vi "gathering.vi"() -> ()   [LabVIEW 2016]
doc: "该模板用于创建生产者／消费者模式的应用程序，以事件驱动的方式，生成队列中的项。如需通过响应事件实现代码的异步执行，同时不影响用户界面的响应速度，可考虑用该模式替代“用户界面事件处理器”模式。"
panel:
  in  "Clear 2":bool
  in  "Clear":bool
  in  "控制选板":enum32{"主界面", "配置界面"}(tab)
  in  "设定压力":dbl
  in  "设定温度":dbl
  out "当前压力":dbl(knob) scale=0.0..10.0
  out "当前温度":dbl(slide) scale=0.0..100.0
  in  "刚度计算":bool
  out "样件结果数据":T1
  in  "自动":bool
  in  "手动":bool
  out "拉伸力":dbl
  in  "弯曲 2":bool caption="元素入队列"
  out "扭矩":dbl
  out "扭转角度2":dbl
  out "弯曲力":dbl
  out "拉伸位移":dbl
  out "扭转角度":dbl
  out "弯曲位移":dbl
  in  "复位3":bool caption="元素入队列"
  in  "拉伸":bool caption="元素入队列"
  in  "停止3":bool
  in  "复位2":bool caption="元素入队列"
  in  "扭转":bool caption="元素入队列"
  in  "停止2":bool
  in  "复位1":bool caption="元素入队列"
  in  "弯曲":bool caption="元素入队列"
  in  "停止1":bool
  out "弯曲":cluster{"Y":dbl[], "Y":dbl[]}[](graph)
  out "扭转":cluster{"Y":dbl[], "Y":dbl[]}[](graph)
  out "扭转刚度":dbl
  out "拉伸刚度":dbl
  out "弯曲刚度二":dbl
  out "弯曲刚度一":dbl
  out "拉伸":cluster{"Y":dbl[], "Y":dbl[]}[](graph)
  out "下行停止状态":bool
  out "下行状态":bool
  out "上行状态":bool
  out "上行停止状态":bool
  out "下行停止状态 2":bool
  out "下行状态 2":bool
  out "上行状态 2":bool
  out "上行停止状态 2":bool
  out "下行停止状态 3":bool
  out "下行状态 3":bool
  out "上行状态 3":bool
  out "上行停止状态 3":bool
  out "弯曲伺服":dbl
  out "扭转伺服":dbl
  out "拉伸伺服":dbl
  in  "设定弯曲行程":dbl=50000.0
  in  "设置弯曲速度":dbl=10000.0
  in  "设定扭转距离":dbl=50000.0
  in  "设置扭转速度":dbl=10000.0
  in  "设定拉升行程":dbl=50000.0
  in  "设置拉伸速度":dbl=10000.0
  in  "automitic":bool
  out "拉伸停止":bool
  out "扭转停止":bool
  out "弯曲停止":bool
  in  "运行状态 3":string
  in  "运行状态 2":string
  out "运行状态":string
  out "弯曲控制采集停止状态":bool
  in  "手动方向":bool
  in  "弯曲计算":string
  out "设备打开成功":bool
  out "私服使能关闭 3":bool
  in  "私服使能 3":bool
  out "改变速度成功 3":bool
  out "轴关闭成功 3":bool
  out "轴打开成功 3":bool
  out "急速停止成功 3":bool
  out "减速停止成功 3":bool
  out "相对运动 3":bool
  out "绝对运动 3":bool
  out "重置计数器成功 3":bool
  out "轴的状态: 3":string
  out "当前指令的速度 3":dbl
  out "私服使能关闭 2":bool
  in  "私服使能 2":bool
  out "改变速度成功 2":bool
  out "轴关闭成功 2":bool
  out "轴打开成功 2":bool
  out "急速停止成功 2":bool
  out "减速停止成功 2":bool
  out "相对运动 2":bool
  out "绝对运动 2":bool
  out "重置计数器成功 2":bool
  out "轴的状态: 2":string
  out "当前指令的速度 2":dbl
  out "当前轴达到最大速度":bool
  out "?":bool
  out "设备关闭成功":bool
  out "轴打开成功":bool
  out "急速停止成功":bool
  out "减速停止成功":bool
  out "重置计数器成功":bool
  in  "停止模式":enum32{"Dec", "Emg"}(radio)
  out "轴的数量":u32
  in  "Device Type":u16(ring) items=["PCI-1285 (M0)"]
  in  "withdraw":bool caption="停止"
  out "deviceList":u32[](array[numeric])
  out "DeviceHandle":u32
  out "AxisHandle_Array":u32[](array[numeric])
  in  "采集卡开关":bool=TRUE caption="stop(true)"
  out "error out":errorcluster
  out "轴的状态:":string
  # "控制状态"
  # "参数设置"
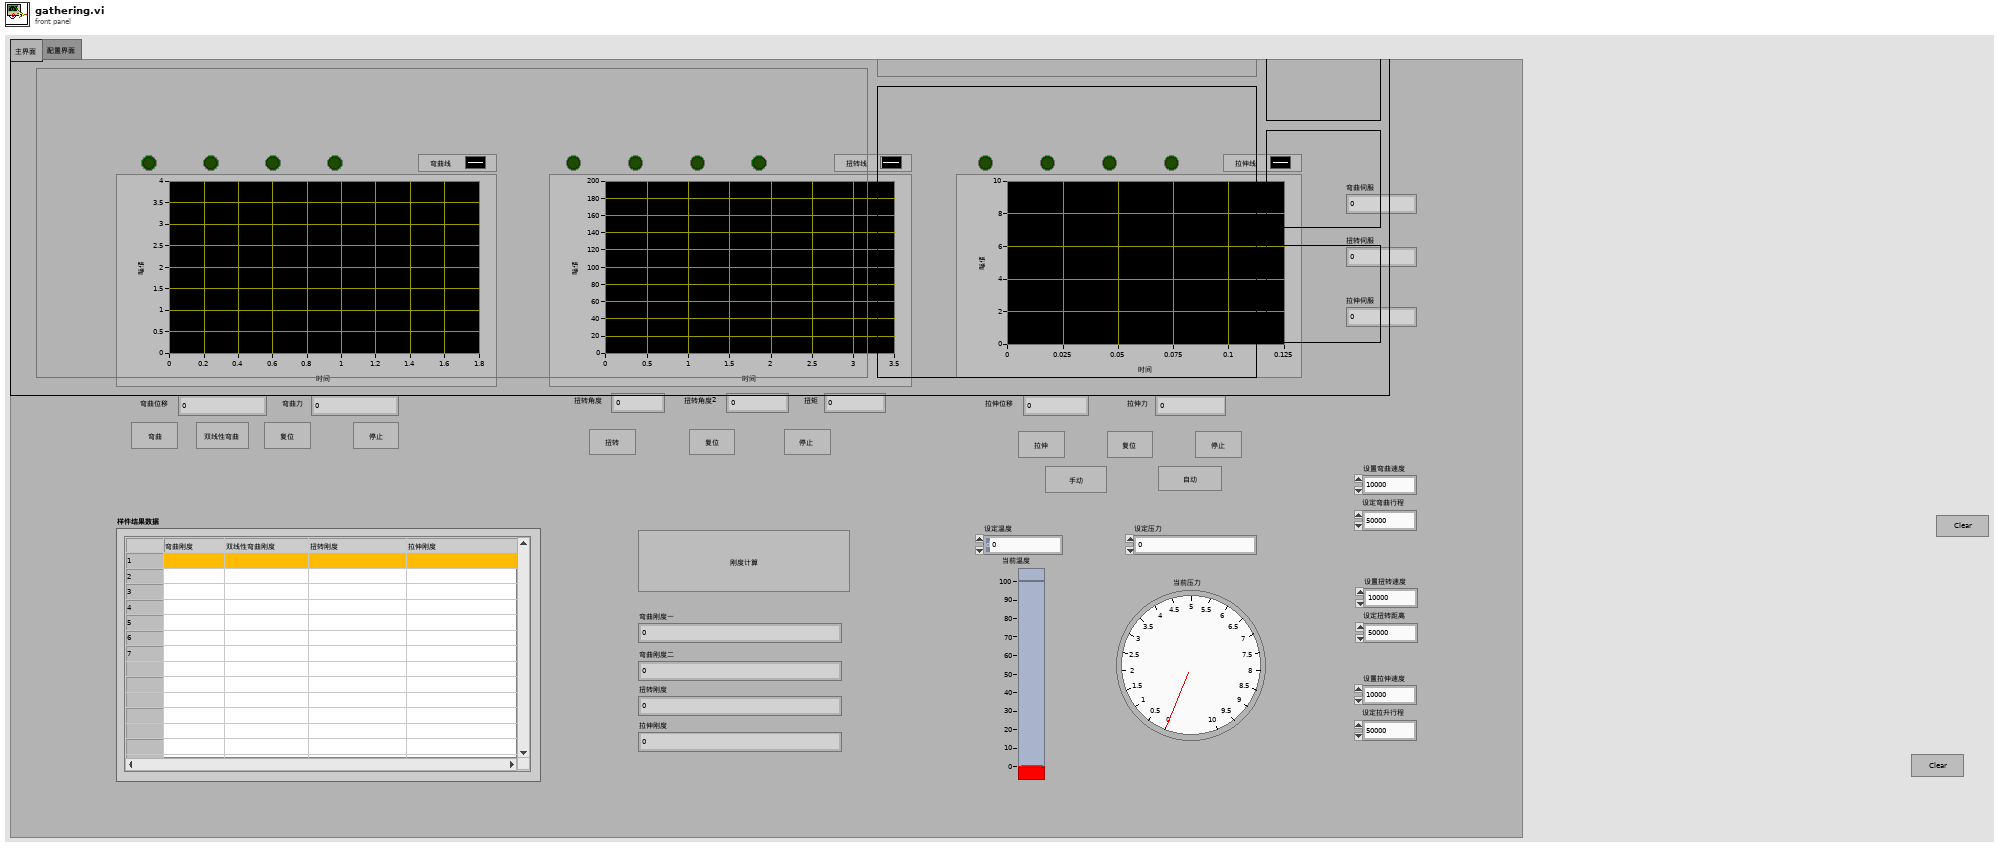
[diagram p1: front panel]
types:
  T1 = typedef "控件 1.ctl" = i32
  T2 = enum16{"open", "replace", "create", "open or create", "replace or create", "replace or create with confirmation"}
  T3 = enum8{"Enabled", "Disabled", "Disabled and Grayed Out"}
  T4 = cluster{"DeviceNum":u32, "U*8 Array":cluster{"U*8 Array[0]":u8, "U*8 Array[1]":u8, "U*8 Array[2]":u8, "U*8 Array[3]":u8, "U*8 Array[4]":u8, "U*8 Array[5]":u8, "U*8 Array[6]":u8, "U*8 Array[7]":u8, "U*8 Array[8]":u8, "U*8 Array[9]":u8, "U*8 Array[10]":u8, "U*8 Array[11]":u8, "U*8 Array[12]":u8, "U*8 Array[13]":u8, "U*8 Array[14]":u8, "U*8 Array[15]":u8, "U*8 Array[16]":u8, "U*8 Array[17]":u8, "U*8 Array[18]":u8, "U*8 Array[19]":u8, "U*8 Array[20]":u8, "U*8 Array[21]":u8, "U*8 Array[22]":u8, "U*8 Array[23]":u8, "U*8 Array[24]":u8, "U*8 Array[25]":u8, "U*8 Array[26]":u8, "U*8 Array[27]":u8, "U*8 Array[28]":u8, "U*8 Array[29]":u8, "U*8 Array[30]":u8, "U*8 Array[31]":u8, "U*8 Array[32]":u8, "U*8 Array[33]":u8, "U*8 Array[34]":u8, "U*8 Array[35]":u8, "U*8 Array[36]":u8, "U*8 Array[37]":u8, "U*8 Array[38]":u8, "U*8 Array[39]":u8, "U*8 Array[40]":u8, "U*8 Array[41]":u8, "U*8 Array[42]":u8, "U*8 Array[43]":u8, "U*8 Array[44]":u8, "U*8 Array[45]":u8, "U*8 Array[46]":u8, "U*8 Array[47]":u8, "U*8 Array[48]":u8, "U*8 Array[49]":u8}, "NumOfSubDevice":i16}[]
  T5 = cluster{"U*8 Array[0]":u8, "U*8 Array[1]":u8, "U*8 Array[2]":u8, "U*8 Array[3]":u8, "U*8 Array[4]":u8, "U*8 Array[5]":u8, "U*8 Array[6]":u8, "U*8 Array[7]":u8, "U*8 Array[8]":u8, "U*8 Array[9]":u8, "U*8 Array[10]":u8, "U*8 Array[11]":u8, "U*8 Array[12]":u8, "U*8 Array[13]":u8, "U*8 Array[14]":u8, "U*8 Array[15]":u8, "U*8 Array[16]":u8, "U*8 Array[17]":u8, "U*8 Array[18]":u8, "U*8 Array[19]":u8, "U*8 Array[20]":u8, "U*8 Array[21]":u8, "U*8 Array[22]":u8, "U*8 Array[23]":u8, "U*8 Array[24]":u8, "U*8 Array[25]":u8, "U*8 Array[26]":u8, "U*8 Array[27]":u8, "U*8 Array[28]":u8, "U*8 Array[29]":u8, "U*8 Array[30]":u8, "U*8 Array[31]":u8, "U*8 Array[32]":u8, "U*8 Array[33]":u8, "U*8 Array[34]":u8, "U*8 Array[35]":u8, "U*8 Array[36]":u8, "U*8 Array[37]":u8, "U*8 Array[38]":u8, "U*8 Array[39]":u8, "U*8 Array[40]":u8, "U*8 Array[41]":u8, "U*8 Array[42]":u8, "U*8 Array[43]":u8, "U*8 Array[44]":u8, "U*8 Array[45]":u8, "U*8 Array[46]":u8, "U*8 Array[47]":u8, "U*8 Array[48]":u8, "U*8 Array[49]":u8}
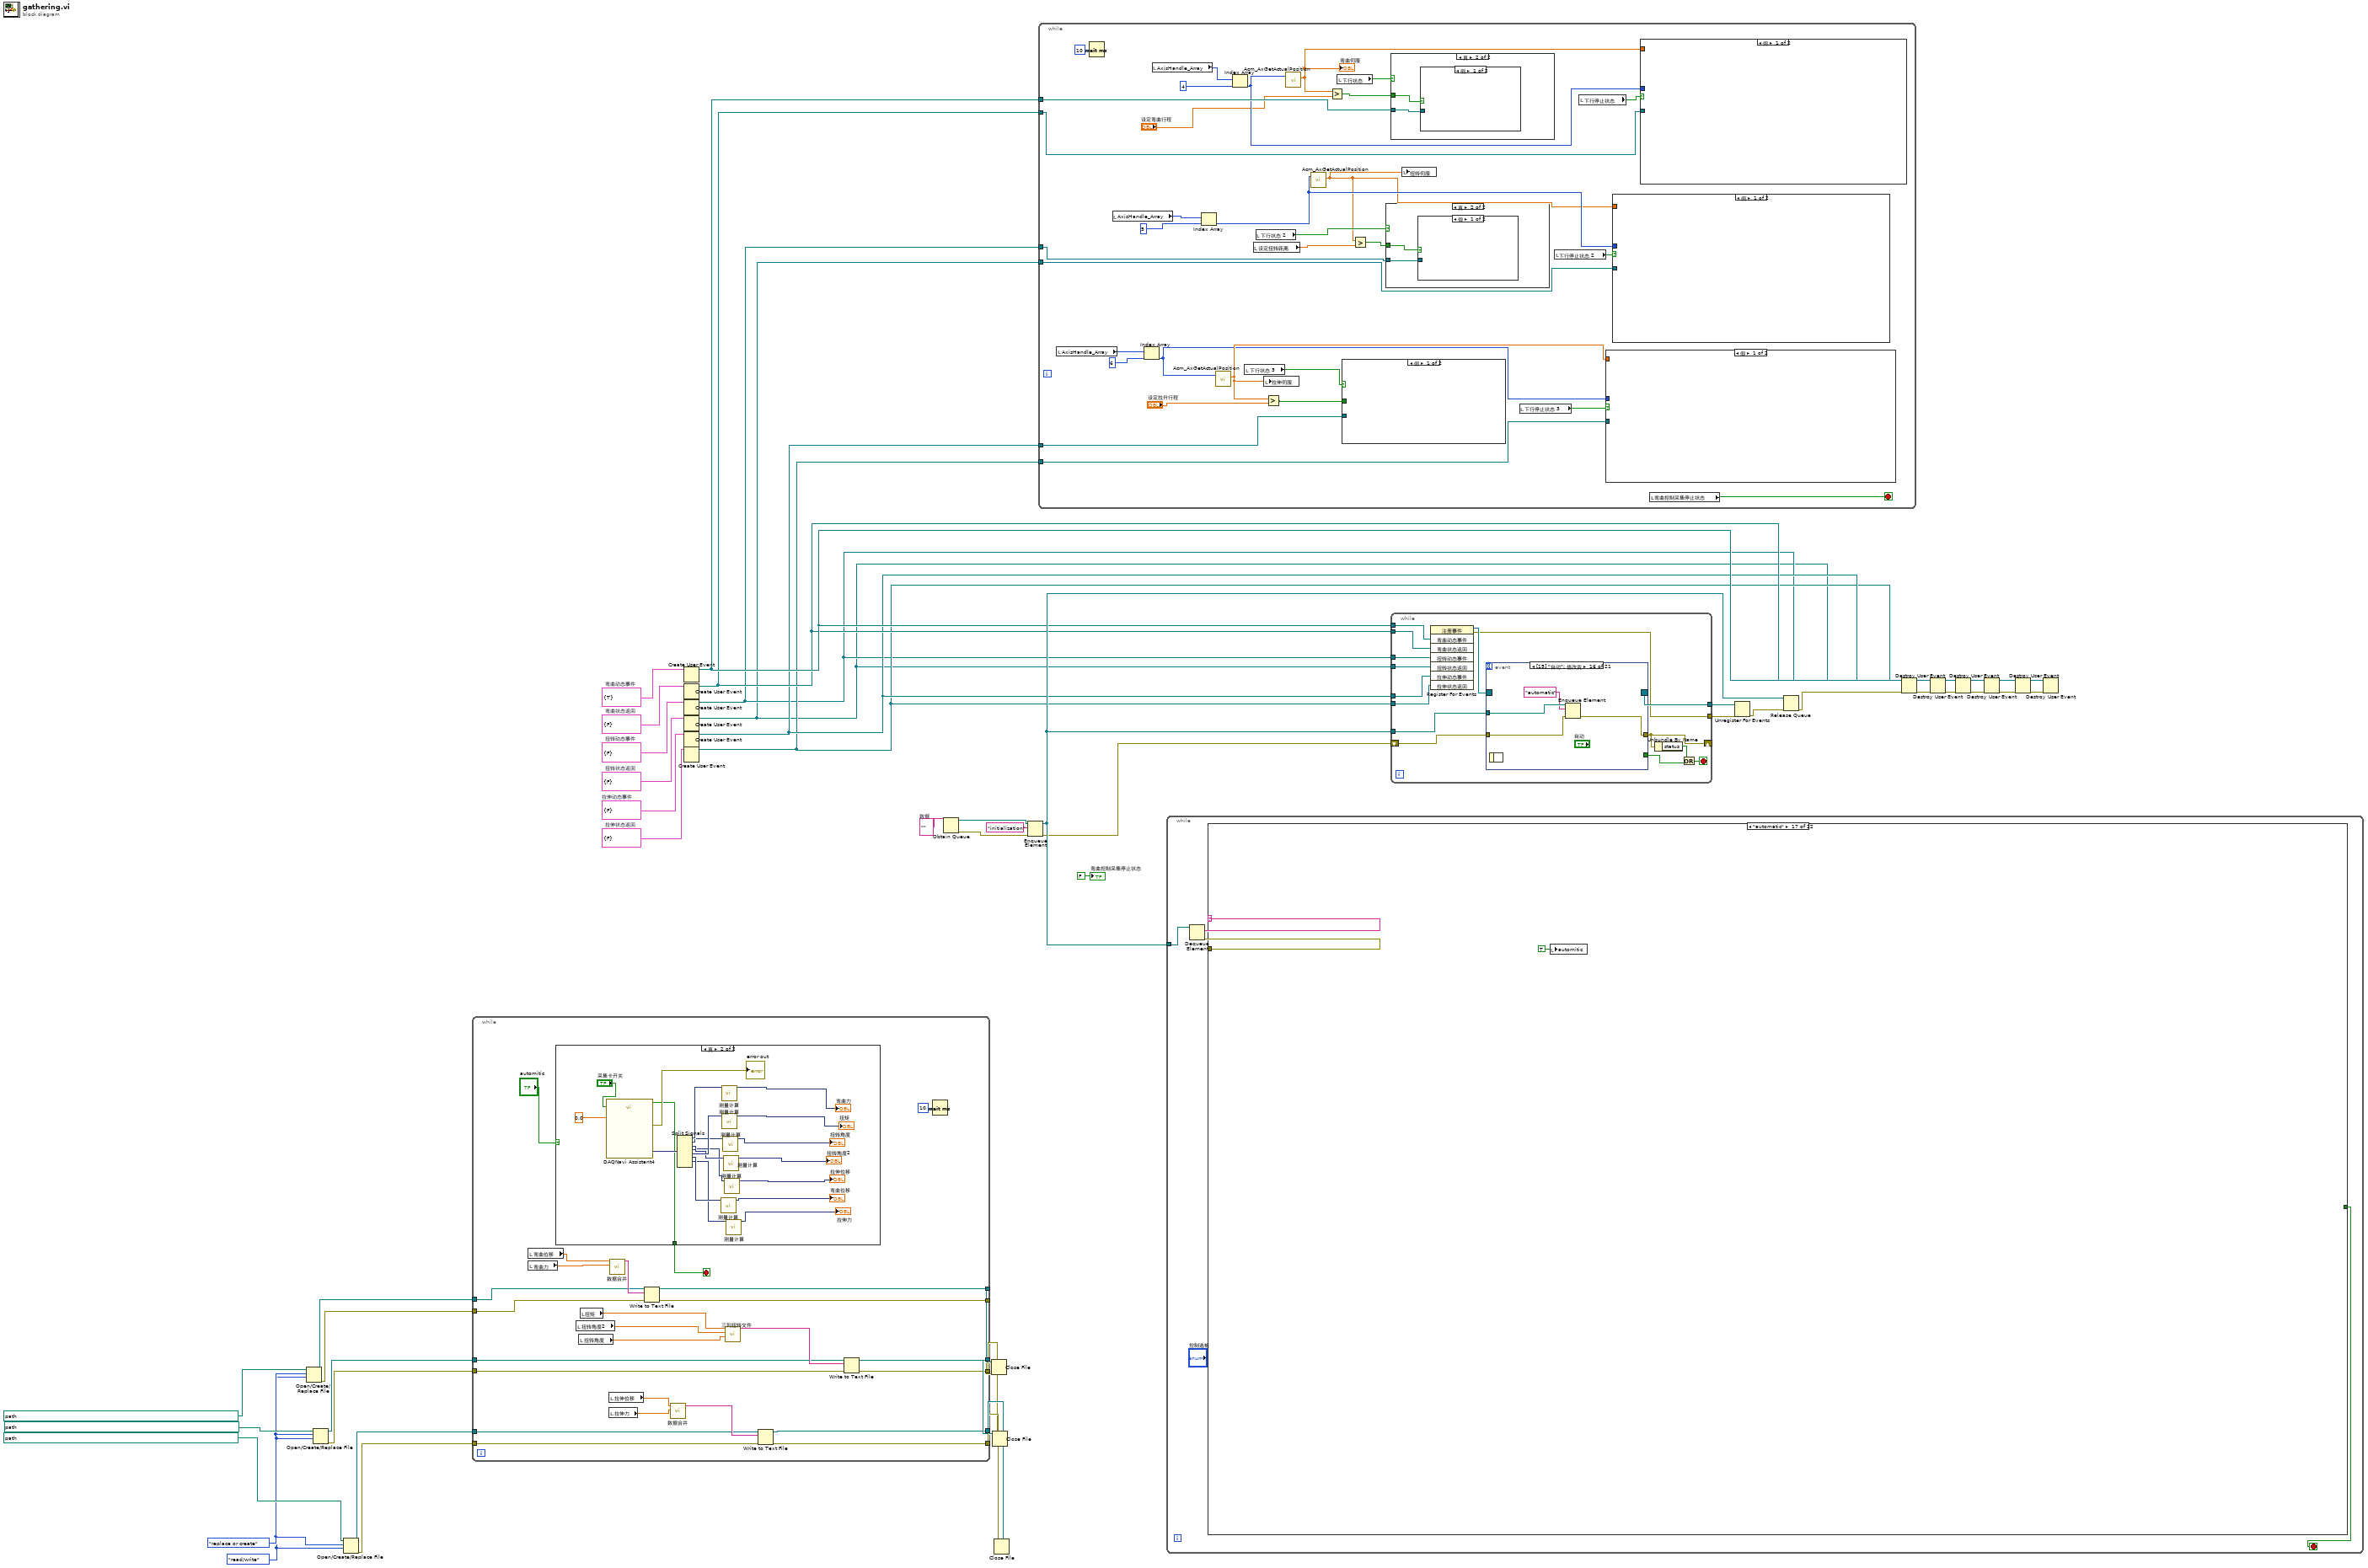
[diagram p0: block diagram]
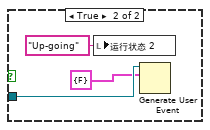
[diagram p3: hidden frame]
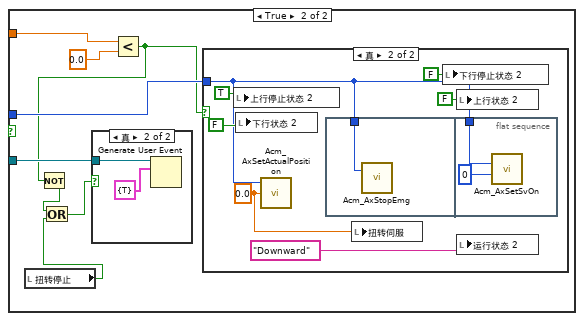
[diagram p4: hidden frame]
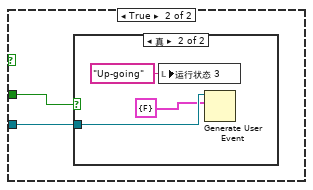
[diagram p7: hidden frame]
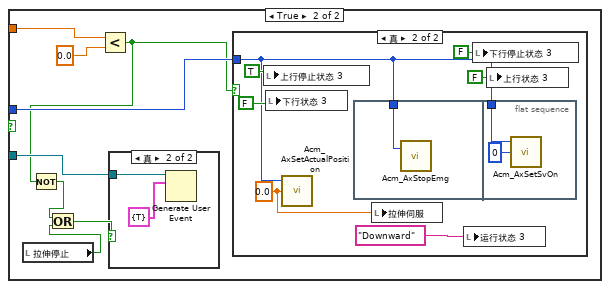
[diagram p9: hidden frame]
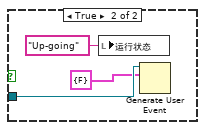
[diagram p13: hidden frame]
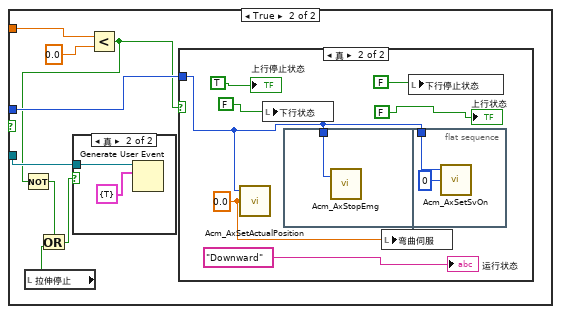
[diagram p14: hidden frame]
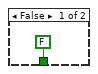
[diagram p17: hidden frame]
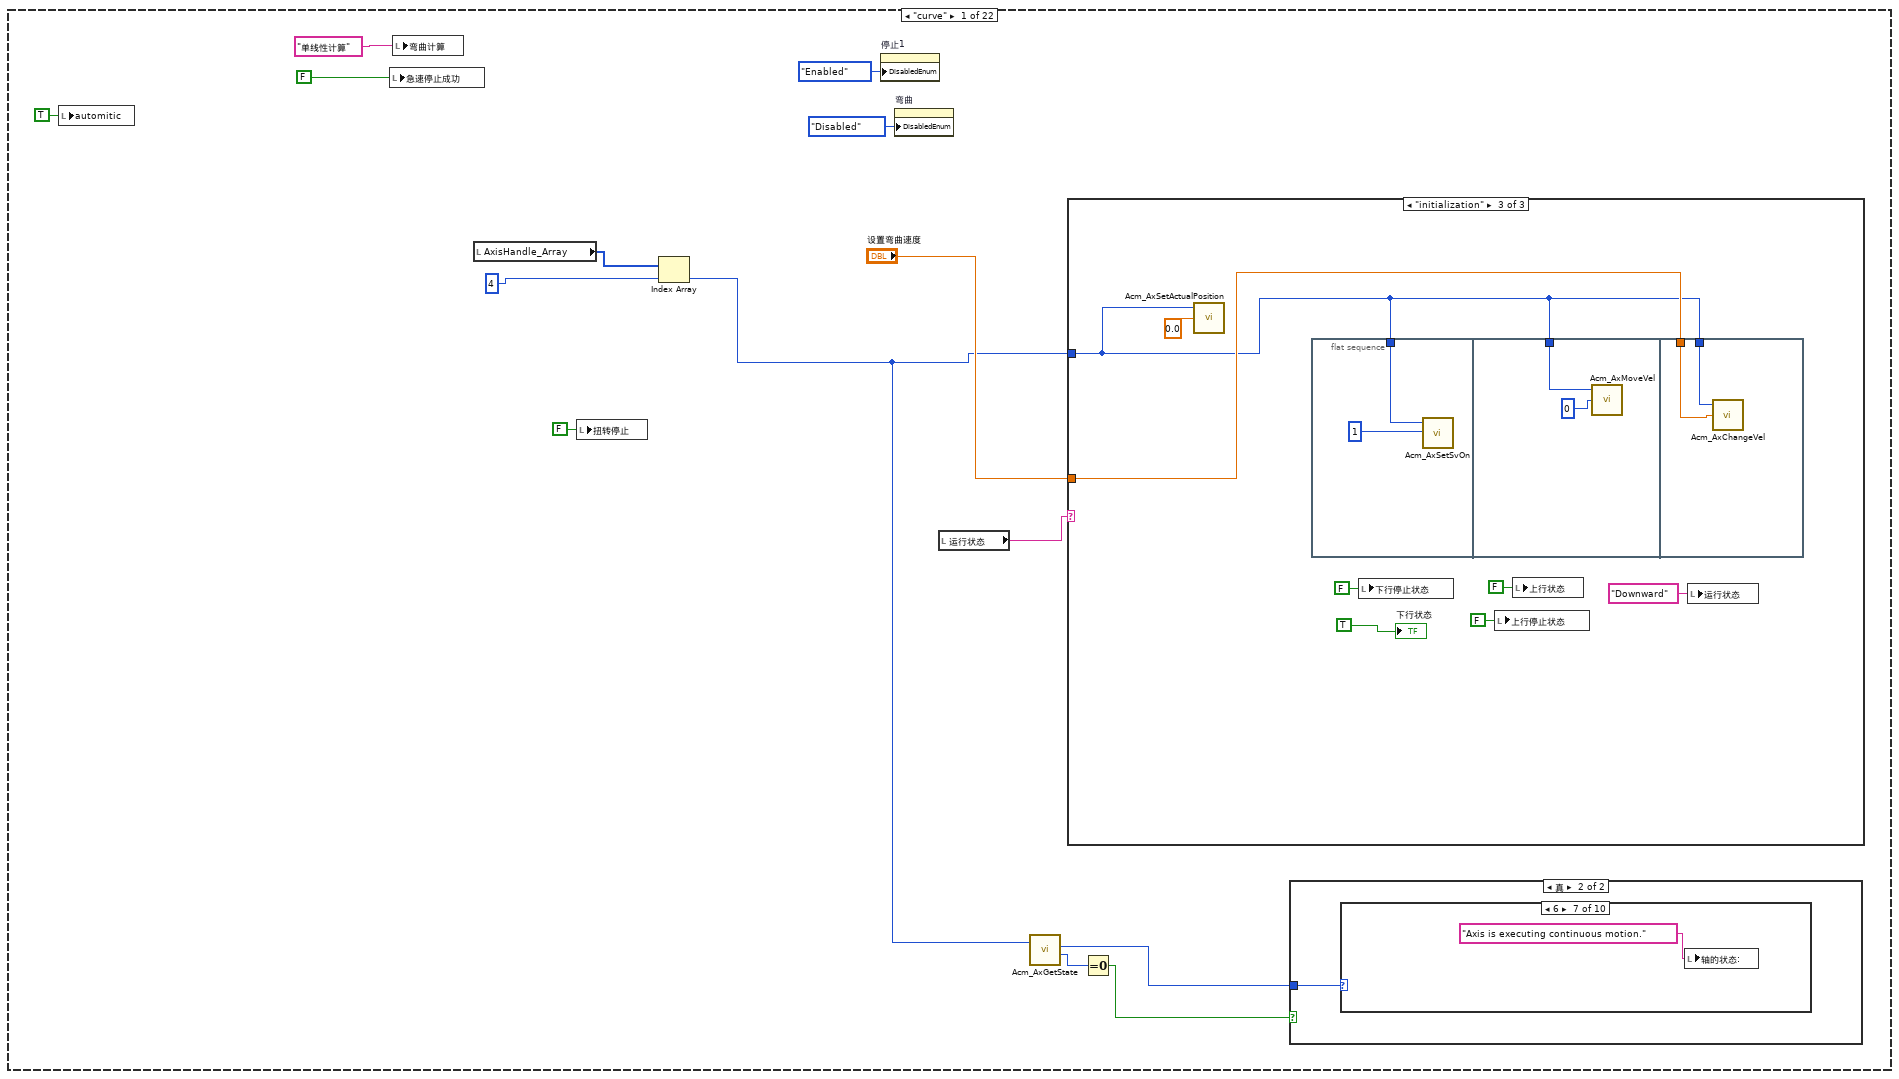
[diagram p18: hidden frame]
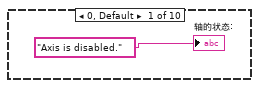
[diagram p20: hidden frame]
diagram:
  w14 = cluster{"拉升状态返回":bool} {"拉升状态返回"=FALSE}  # 拉伸状态返回
  w13 = cluster{"拉伸动态事件":bool} {"拉伸动态事件"=FALSE}  # 拉伸动态事件
  w12 = cluster{"扭转状态返回":bool} {"扭转状态返回"=FALSE}  # 扭转状态返回
  w11 = cluster{"扭转动态事件":bool} {"扭转动态事件"=FALSE}  # 扭转动态事件
  w16 = cluster{"弯曲状态返回":bool} {"弯曲状态返回"=FALSE}  # 弯曲状态返回
  w19 = cluster{"弯曲动态触发":bool} {"弯曲动态触发"=TRUE}  # 弯曲动态事件
  w33 = enum16{"read/write", "read-only", "write-only"}."read/write" ("权限(0:read/write)")
  w34 = T2."replace or create" ("操作(0:open)")
  w45 = ""  # 数据
  n1 = Open/Create/Replace File(file path (use dialog)=path "D:/controller/for_test_line/test_line/Collecting polymorphism/弯曲刚度检测数据.txt" ("文件路径（使用对话框）"), operation (0:open)=w34, access (0:read/write)=w33) -> (refnum out=w32:refnum<file>, error out=w31:errorcluster)  [unwired: 3 in, 1 out]
  n2 = Open/Create/Replace File(file path (use dialog)=path "D:/controller/for_test_line/test_line/Collecting polymorphism/扭转刚度检测数据.txt" ("文件路径（使用对话框）"), operation (0:open)=w34, access (0:read/write)=w33) -> (refnum out=w39:refnum<file>, error out=w38:errorcluster)  [unwired: 3 in, 1 out]
  n3 = Open/Create/Replace File(file path (use dialog)=path "D:/controller/for_test_line/test_line/Collecting polymorphism/拉伸刚度检测数据.txt" ("文件路径（使用对话框）"), operation (0:open)=w34, access (0:read/write)=w33) -> (refnum out=w37:refnum<file>, error out=w36:errorcluster)  [unwired: 3 in, 1 out]
  n4 = while {
    tunnel: w39 -> [w57]
    tunnel: w38 -> [w56]
    tunnel: w37 -> [w67]
    tunnel: w36 -> [w66]
    tunnel: w32 -> [w52]
    tunnel: w31 -> [w51]
    tunnel: [w65] -> w30
    tunnel: [w64] -> w29
    tunnel: [w54] -> w28
    tunnel: [w53] -> w27
    tunnel: [w50] -> w26
    tunnel: [w49] -> w25
    stop <- w46 stop-if-true
    n5 = local read "弯曲位移"() -> (w59:dbl)
    n6 = local read "弯曲力"() -> (w60:dbl)
    n7 = case shown="真" "automitic" {
      tunnel: [FALSE ("stopped") w72] -> w46
      frame False {
      }
      frame True {
        n8 = call "DAQNavi Assistant4"("stop(true)"="采集卡开关", "conversion rate(Hz)"=0.0) -> ("error out"=→"error out":errorcluster, "data out(DDT)"=w85:dynamicdata, "stopped"=w72:bool)  [unwired: 4 in, 19 out]
        n9 = Split Signals(w85) -> (w81:dynamicdata, w79:dynamicdata, w78:dynamicdata, w77:dynamicdata, w80:dynamicdata, w75:dynamicdata, w74:dynamicdata)  [unwired: 8 in, 1 out]
        n10 = call "测量计算.vi"("Dynamic Data输入"=w75) -> ("Dynamic Data输出"=→"弯曲位移":dynamicdata)  [unwired: 10 in]
        n11 = call "测量计算.vi"("Dynamic Data输入"=w81) -> ("Dynamic Data输出"=→"弯曲力":dynamicdata)  [unwired: 10 in]
        n12 = call "测量计算.vi"("Dynamic Data输入"=w80) -> ("Dynamic Data输出"=→"扭矩":dynamicdata)  [unwired: 10 in]
        n13 = call "测量计算.vi"("Dynamic Data输入"=w79) -> ("Dynamic Data输出"=→"扭转角度":dynamicdata)  [unwired: 10 in]
        n14 = call "测量计算.vi"("Dynamic Data输入"=w78) -> ("Dynamic Data输出"=→"扭转角度2":dynamicdata)  [unwired: 10 in]
        n15 = call "测量计算.vi"("Dynamic Data输入"=w77) -> ("Dynamic Data输出"=→"拉伸位移":dynamicdata)  [unwired: 10 in]
        n16 = call "测量计算.vi"("Dynamic Data输入"=w74) -> ("Dynamic Data输出"=→"拉伸力":dynamicdata)  [unwired: 10 in]
      }
    }
    n17 = local read "扭转角度2"() -> (w62:dbl)
    n18 = local read "扭转角度"() -> (w61:dbl)
    n19 = local read "扭矩"() -> (w63:dbl)
    n20 = local read "拉伸位移"() -> (w69:dbl)
    n21 = local read "拉伸力"() -> (w70:dbl)
    n22 = call "数据合并.vi"("数值输入"=w60, "数值 3"=w59) -> ("字符串"=w55:string)  [unwired: 9 in]
    n23 = Write to Text File(file (use dialog)=w52, text=w55, error in=w51) -> (refnum out=w50:refnum<file>, error out=w49:errorcluster)  [unwired: 1 in, 1 out]
    n24 = call "数据合并.vi"("数值输入"=w70, "数值 3"=w69) -> ("字符串"=w68:string)  [unwired: 9 in]
    n25 = call "三列扭转文件.vi"("扭转角度"=w61, "扭转角度2"=w62, "扭矩"=w63) -> ("字符串"=w58:string)  [unwired: 8 in]
    n26 = Write to Text File(file (use dialog)=w67, text=w68, error in=w66) -> (refnum out=w65:refnum<file>, error out=w64:errorcluster)  [unwired: 1 in, 1 out]
    n27 = Write to Text File(file (use dialog)=w57, text=w58, error in=w56) -> (refnum out=w54:refnum<file>, error out=w53:errorcluster)  [unwired: 1 in, 1 out]
    n28 = Wait (ms)(milliseconds to wait=u32 10 ("等待时间（毫秒）")) -> ()  [unwired: 1 out]
  }
  n29 = Create User Event(user event datatype=w19) -> (user event=w20:refnum<user-event>)  [unwired: 1 in, 1 out]
  n30 = Create User Event(user event datatype=w16) -> (user event=w17:refnum<user-event>)  [unwired: 1 in, 1 out]
  n31 = Create User Event(user event datatype=w11) -> (user event=w4:refnum<user-event>)  [unwired: 1 in, 1 out]
  n32 = Create User Event(user event datatype=w12) -> (user event=w3:refnum<user-event>)  [unwired: 1 in, 1 out]
  n33 = Create User Event(user event datatype=w13) -> (user event=w6:refnum<user-event>)  [unwired: 1 in, 1 out]
  n34 = Create User Event(user event datatype=w14) -> (user event=w5:refnum<user-event>)  [unwired: 1 in, 1 out]
  n35 = Obtain Queue(element data type=w45) -> (queue out=w44:refnum<queue>, error out=w43:errorcluster)  [unwired: 4 in, 1 out]
  n36 = Close File(refnum=w26, error in=w25) -> ()  [unwired: 2 out]
  n37 = Close File(refnum=w28, error in=w27) -> ()  [unwired: 2 out]
  n38 = Close File(refnum=w30, error in=w29) -> ()  [unwired: 2 out]
  n39 = Enqueue Element(queue=w44, element="initialization" ("元素"), error in (no error)=w43) -> (queue out=w24:refnum<queue>, error out=w15:errorcluster)  [unwired: 1 in, 1 out]
  n40 = while "While循环" {
    tunnel: w20 -> [w119]
    tunnel: w17 -> [w117]
    tunnel: w6 -> [w106]
    tunnel: w5 -> [w105]
    tunnel: w4 -> [w96]
    tunnel: w3 -> [w95]
    stop <- w120 stop-if-true
    # "弯曲位置采集"
    n41 = local read "AxisHandle_Array"() -> (w108:u32[])
    n42 = Wait (ms)(milliseconds to wait=u32 10 ("等待时间（毫秒）")) -> ()  [unwired: 1 out]
    n43 = local read "AxisHandle_Array"() -> (w103:u32[])
    n44 = Index Array(array=w108, index=6 ("索引")) -> (element=w110:u32)
    n45 = local read "AxisHandle_Array"() -> (w121:u32[])
    n46 = Index Array(array=w103, index=5 ("索引")) -> (element=w101:u32)
    n47 = call <userlib>:"Acm_AxGetActualPosition.vi"("AxisHandle"=w110) -> ("Position"=w112:dbl)  [unwired: 1 in, 3 out]
    n48 = Index Array(array=w121, index=4 ("索引")) -> (element=w116:u32)
    n49 = local read "下行状态 3"() -> (w111:bool)
    n50 = local read "设定扭转距离"() -> (w98:dbl)
    n51 = local read "下行状态 2"() -> (w100:bool)
    n52 = local write "拉伸伺服"(w112) -> ()
    n53 = Greater?(x=w112, y="设定拉升行程") -> (0:w113:bool)
    n54 = call <userlib>:"Acm_AxGetActualPosition.vi"("AxisHandle"=w116) -> ("Position"=w91:dbl)  [unwired: 1 in, 3 out]
    "弯曲伺服" <- w91
    n55 = call <userlib>:"Acm_AxGetActualPosition.vi"("AxisHandle"=w101) -> ("Position"=w99:dbl)  [unwired: 1 in, 3 out]
    n56 = Greater?(x=w91, y="设定弯曲行程") -> (0:w114:bool)
    n57 = local read "下行状态"() -> (w115:bool)
    n58 = case shown="假" w111 {
      tunnel: w113 -> [_ w149]
      tunnel: w106 -> [_ w148]
      frame False {
      }
      frame True {
        n59 = case shown="真" w149 {
          tunnel: w148 -> [_ w152]
          frame False {
          }
          frame True {
            n60 = local write "运行状态 3"("Up-going" ("运行状态")) -> ()
            n61 = Generate User Event(user event=w152, event data cluster=cluster{"弯曲动态触发":bool} {"弯曲动态触发"=FALSE} ("事件数据")) -> ()  [unwired: 2 in, 2 out]
          }
        }
      }
    }
    n62 = Greater?(x=w99, y=w98) -> (0:w97:bool)
    n63 = case shown="真" w100 {
      tunnel: w97 -> [_ w124]
      tunnel: w96 -> [_ w123]
      frame False {
      }
      frame True {
        n64 = case shown="假" w124 {
          tunnel: w123 -> [_ w127]
          frame False {
          }
          frame True {
            n65 = local write "运行状态 2"("Up-going" ("运行状态")) -> ()
            n66 = Generate User Event(user event=w127, event data cluster=cluster{"弯曲动态触发":bool} {"弯曲动态触发"=FALSE} ("事件数据")) -> ()  [unwired: 2 in, 2 out]
          }
        }
      }
    }
    n67 = case shown="真" w115 {
      tunnel: w114 -> [_ w174]
      tunnel: w119 -> [_ w173]
      frame False {
      }
      frame True {
        n68 = case shown="假" w174 {
          tunnel: w173 -> [_ w177]
          frame False {
          }
          frame True {
            n69 = local write "运行状态"("Up-going" ("运行状态")) -> ()
            n70 = Generate User Event(user event=w177, event data cluster=cluster{"弯曲动态触发":bool} {"弯曲动态触发"=FALSE} ("事件数据")) -> ()  [unwired: 2 in, 2 out]
          }
        }
      }
    }
    n71 = local write "扭转伺服"(w99) -> ()
    n72 = local read "下行停止状态 3"() -> (w109:bool)
    n73 = local read "下行停止状态 2"() -> (w102:bool)
    n74 = local read "下行停止状态"() -> (w118:bool)
    n75 = case shown="假" w109 {
      tunnel: w105 -> [_ w160]
      tunnel: w112 -> [_ w159]
      tunnel: w110 -> [_ w157]
      frame False {
      }
      frame True {
        n76 = local read "拉伸停止"() -> (w154:bool)
        n77 = Less?(x=w159, y=0.0) -> (x < y?=w156:bool)
        n78 = Not(x=w156) -> (.not. x?=w155:bool)
        n79 = Or(x=w155, y=w154) -> (x .or. y?=w153:bool)
        n80 = case shown="真" w153 {
          tunnel: w160 -> [_ w162]
          frame False {
          }
          frame True {
            n81 = Generate User Event(user event=w162, event data cluster=cluster{"弯曲动态触发":bool} {"弯曲动态触发"=TRUE} ("事件数据")) -> ()  [unwired: 2 in, 2 out]
          }
        }
        n82 = case shown="真" w156 {
          tunnel: w157 -> [_ w165]
          frame False {
          }
          frame True {
            w164 = 0.0 ("Position")
            n83 = local write "上行停止状态 3"(TRUE ("上行停止状态")) -> ()
            n84 = local write "下行状态 3"(FALSE ("下行状态")) -> ()
            n85 = call <userlib>:"Acm_AxSetActualPosition.vi"("Position"=w164, "AxisHandle"=w165) -> ()  [unwired: 1 in, 3 out]
            n86 = flat-sequence {
              tunnel: w165 -> [w170]
              tunnel: w165 -> [w172]
              frame #0 {
                n87 = call <userlib>:"Acm_AxStopEmg.vi"("AxisHandle"=w170) -> ()  [unwired: 1 in, 3 out]
              }
              frame #1 {
                n88 = call <userlib>:"Acm_AxSetSvOn.vi"("OnOff"=u32 0, "AxisHandle"=w172) -> ()  [unwired: 1 in, 3 out]
              }
            }
            n89 = local write "拉伸伺服"(w164) -> ()
            n90 = local write "运行状态 3"("Downward" ("运行状态 3")) -> ()
            n91 = local write "下行停止状态 3"(FALSE ("下行停止状态")) -> ()
            n92 = local write "上行状态 3"(FALSE ("上行状态")) -> ()
          }
        }
      }
    }
    n93 = case shown="假" w102 {
      tunnel: w95 -> [_ w135]
      tunnel: w99 -> [_ w134]
      tunnel: w101 -> [_ w132]
      frame False {
      }
      frame True {
        n94 = local read "扭转停止"() -> (w130:bool)
        n95 = Less?(x=w134, y=0.0) -> (x < y?=w131:bool)
        n96 = Not(x=w131) -> (.not. x?=w129:bool)
        n97 = Or(x=w129, y=w130) -> (x .or. y?=w128:bool)
        n98 = case shown="真" w128 {
          tunnel: w135 -> [_ w137]
          frame False {
          }
          frame True {
            n99 = Generate User Event(user event=w137, event data cluster=cluster{"弯曲动态触发":bool} {"弯曲动态触发"=TRUE} ("事件数据")) -> ()  [unwired: 2 in, 2 out]
          }
        }
        n100 = case shown="真" w131 {
          tunnel: w132 -> [_ w140]
          frame False {
          }
          frame True {
            w139 = 0.0 ("Position")
            n101 = local write "上行停止状态 2"(TRUE ("上行停止状态")) -> ()
            n102 = local write "下行状态 2"(FALSE ("下行状态")) -> ()
            n103 = call <userlib>:"Acm_AxSetActualPosition.vi"("Position"=w139, "AxisHandle"=w140) -> ()  [unwired: 1 in, 3 out]
            n104 = flat-sequence {
              tunnel: w140 -> [w145]
              tunnel: w140 -> [w147]
              frame #0 {
                n105 = call <userlib>:"Acm_AxStopEmg.vi"("AxisHandle"=w145) -> ()  [unwired: 1 in, 3 out]
              }
              frame #1 {
                n106 = call <userlib>:"Acm_AxSetSvOn.vi"("OnOff"=u32 0, "AxisHandle"=w147) -> ()  [unwired: 1 in, 3 out]
              }
            }
            n107 = local write "扭转伺服"(w139) -> ()
            n108 = local write "下行停止状态 2"(FALSE ("下行停止状态")) -> ()
            n109 = local write "上行状态 2"(FALSE ("上行状态")) -> ()
            n110 = local write "运行状态 2"("Downward" ("运行状态 2")) -> ()
          }
        }
      }
    }
    n111 = case shown="假" w118 {
      tunnel: w117 -> [_ w185]
      tunnel: w91 -> [_ w184]
      tunnel: w116 -> [_ w182]
      frame False {
      }
      frame True {
        n112 = local read "拉伸停止"() -> (w180:bool)
        n113 = Less?(x=w184, y=0.0) -> (x < y?=w181:bool)
        n114 = Not(x=w181) -> (.not. x?=w179:bool)
        n115 = Or(x=w179, y=w180) -> (x .or. y?=w178:bool)
        n116 = case shown="真" w178 {
          tunnel: w185 -> [_ w187]
          frame False {
          }
          frame True {
            n117 = Generate User Event(user event=w187, event data cluster=cluster{"弯曲动态触发":bool} {"弯曲动态触发"=TRUE} ("事件数据")) -> ()  [unwired: 2 in, 2 out]
          }
        }
        n118 = case shown="真" w181 {
          tunnel: w182 -> [_ w192]
          frame False {
          }
          frame True {
            w191 = 0.0 ("Position")
            n119 = call <userlib>:"Acm_AxSetActualPosition.vi"("Position"=w191, "AxisHandle"=w192) -> ()  [unwired: 1 in, 3 out]
            n120 = local write "下行状态"(FALSE ("下行状态")) -> ()
            n121 = flat-sequence {
              tunnel: w192 -> [w195]
              tunnel: w192 -> [w197]
              frame #0 {
                n122 = call <userlib>:"Acm_AxStopEmg.vi"("AxisHandle"=w195) -> ()  [unwired: 1 in, 3 out]
              }
              frame #1 {
                n123 = call <userlib>:"Acm_AxSetSvOn.vi"("OnOff"=u32 0, "AxisHandle"=w197) -> ()  [unwired: 1 in, 3 out]
              }
            }
            n124 = local write "弯曲伺服"(w191) -> ()
            n125 = local write "下行停止状态"(FALSE ("下行停止状态")) -> ()
            "运行状态" <- "Downward" ("运行状态")
            "上行状态" <- FALSE ("上行状态")
            "上行停止状态" <- TRUE ("上行停止状态")
          }
        }
      }
    }
    n126 = local read "弯曲控制采集停止状态"() -> (w120:bool)
  }
  n127 = while {
    tunnel: w24 -> [w201]
    stop <- w200 stop-if-true
    n128 = Dequeue Element(queue=w201) -> (element=w199:string, error out=w198:errorcluster)  [unwired: 2 in, 2 out]
    n129 = case shown="\"automatic\"" w199 {
      tunnel: [_ _ _ _ FALSE ("status") _ _ _ _ _ _ _ _ _ _ _ _ _ _ _ w873 w909] -> w200
      tunnel: w198 -> [_ _ _ _ _ _ _ _ _ _ _ _ _ _ _ _ _ _ _ _ w875 w911]
      frame "curve" {
        n130 = local write "automitic"(TRUE ("automitic")) -> ()
        n131 = local write "急速停止成功"(FALSE ("急速停止成功")) -> ()
        n132 = local write "弯曲计算"("单线性计算" ("采集状态")) -> ()
        n133 = local read "AxisHandle_Array"() -> (w214:u32[])
        n134 = local write "扭转停止"(FALSE ("扭转停止")) -> ()
        n135 = Index Array(array=w214, index=4 ("索引")) -> (element=w206:u32)
        n136 = property on="停止1" class="Bool"("DisabledEnum"=T3."Enabled" ("禁用")) -> ()  [unwired: 2 in, 2 out]
        n137 = property on="弯曲" class="Bool"("DisabledEnum"=T3."Disabled" ("禁用")) -> ()  [unwired: 2 in, 2 out]
        n138 = local read "运行状态"() -> (w211:string)
        n139 = call <userlib>:"Acm_AxGetState.vi"("AxisHandle"=w206) -> ("ReturnValue"=w210:u32, "Status"=w208:u16)  [unwired: 1 in, 2 out]
        n140 = case shown="\"initialization\"" w211 {
          tunnel: w206 -> [w229 w242 w253]
          tunnel: "设置弯曲速度" -> [w228 w241 w260]
          frame "Downward", Default {
            n141 = flat-sequence {
              tunnel: w229 -> [w234]
              tunnel: w229 -> [w237]
              tunnel: w229 -> [w239]
              tunnel: w228 -> [w238]
              frame #0 {
                n142 = call <userlib>:"Acm_AxSetSvOn.vi"("OnOff"=u32 1, "AxisHandle"=w234) -> ()  [unwired: 1 in, 3 out]
              }
              frame #1 {
                n143 = call <userlib>:"Acm_AxMoveVel.vi"("Direction"=u16 0, "AxisHandle"=w237) -> ()  [unwired: 1 in, 3 out]
              }
              frame #2 {
                n144 = call <userlib>:"Acm_AxChangeVel.vi"("NewVelocity"=w238, "AxisHandle"=w239) -> ()  [unwired: 1 in, 3 out]
              }
            }
            n145 = local write "下行停止状态"(FALSE ("下行停止状态")) -> ()
            n146 = local write "下行状态"(TRUE ("下行状态")) -> ()
            n147 = local write "上行停止状态"(FALSE ("上行停止状态")) -> ()
            n148 = local write "上行状态"(FALSE ("上行状态")) -> ()
            n149 = local write "运行状态"("Downward" ("运行状态")) -> ()
          }
          frame "Up-going" {
            n150 = flat-sequence {
              tunnel: w242 -> [w247]
              tunnel: w242 -> [w249]
              tunnel: w242 -> [w252]
              tunnel: w241 -> [w251]
              frame #0 {
                n151 = call <userlib>:"Acm_AxSetSvOn.vi"("OnOff"=u32 1, "AxisHandle"=w247) -> ()  [unwired: 1 in, 3 out]
              }
              frame #1 {
                n152 = call <userlib>:"Acm_AxMoveVel.vi"("Direction"=u16 1, "AxisHandle"=w249) -> ()  [unwired: 1 in, 3 out]
              }
              frame #2 {
                n153 = call <userlib>:"Acm_AxChangeVel.vi"("NewVelocity"=w251, "AxisHandle"=w252) -> ()  [unwired: 1 in, 3 out]
              }
            }
            n154 = local write "下行停止状态"(TRUE ("下行停止状态")) -> ()
            n155 = local write "下行状态"(FALSE ("下行状态")) -> ()
            n156 = local write "上行状态"(TRUE ("上行状态")) -> ()
            n157 = local write "上行停止状态"(FALSE ("上行停止状态")) -> ()
            n158 = local write "运行状态"("Up-going" ("运行状态")) -> ()
          }
          frame "initialization" {
            n159 = call <userlib>:"Acm_AxSetActualPosition.vi"("Position"=0.0, "AxisHandle"=w253) -> ()  [unwired: 1 in, 3 out]
            n160 = flat-sequence {
              tunnel: w253 -> [w261]
              tunnel: w253 -> [w263]
              tunnel: w253 -> [w266]
              tunnel: w260 -> [w265]
              frame #0 {
                n161 = call <userlib>:"Acm_AxSetSvOn.vi"("OnOff"=u32 1, "AxisHandle"=w261) -> ()  [unwired: 1 in, 3 out]
              }
              frame #1 {
                n162 = call <userlib>:"Acm_AxMoveVel.vi"("Direction"=u16 0, "AxisHandle"=w263) -> ()  [unwired: 1 in, 3 out]
              }
              frame #2 {
                n163 = call <userlib>:"Acm_AxChangeVel.vi"("NewVelocity"=w265, "AxisHandle"=w266) -> ()  [unwired: 1 in, 3 out]
              }
            }
            n164 = local write "下行停止状态"(FALSE ("下行停止状态")) -> ()
            n165 = local write "上行停止状态"(FALSE ("上行停止状态")) -> ()
            n166 = local write "上行状态"(FALSE ("上行状态")) -> ()
            n167 = local write "运行状态"("Downward" ("运行状态")) -> ()
            "下行状态" <- TRUE ("下行状态")
          }
        }
        n168 = Equal To 0?(x=w210) -> (x = 0?=w207:bool)
        n169 = case shown="真" w207 {
          tunnel: w208 -> [_ w216]
          frame False {
          }
          frame True {
            n170 = case shown="6" w216 {
              frame 0, Default {
                "轴的状态:" <- "Axis is disabled." ("Axis State:")
              }
              frame 1 {
                n171 = local write "轴的状态:"("Axis is ready." ("Axis State:")) -> ()
              }
              frame 2 {
                n172 = local write "轴的状态:"("Axis is stopping." ("Axis State:")) -> ()
              }
              frame 3 {
                n173 = local write "轴的状态:"("Axis is Error_Stopped." ("Axis State:")) -> ()
              }
              frame 4 {
                n174 = local write "轴的状态:"("Axis is executing home motion." ("Axis State:")) -> ()
              }
              frame 5 {
                n175 = local write "轴的状态:"("Axis is executing PTP motion." ("Axis State:")) -> ()
              }
              frame 6 {
                n176 = local write "轴的状态:"("Axis is executing continuous motion." ("Axis State:")) -> ()
              }
              frame 7 {
                n177 = local write "轴的状态:"("Axis is in Group interpolation motion." ("Axis State:")) -> ()
              }
              frame 8 {
                n178 = local write "轴的状态:"("Axis is executing JOG mode motion." ("Axis State:")) -> ()
              }
              frame 9 {
                n179 = local write "轴的状态:"("Axis is executing MPG mode motion." ("Axis State:")) -> ()
              }
            }
          }
        }
      }
      frame "Curve_stop" {
        n180 = local write "automitic"(TRUE ("automitic")) -> ()
        n181 = local read "停止模式"() -> (w273:enum32{"Dec", "Emg"})
        n182 = local read "AxisHandle_Array"() -> (w275:u32[])
        n183 = Index Array(array=w275, index=4 ("索引")) -> (element=w272:u32)
        n184 = case shown="\"Dec\", 默认" w273 {
          tunnel: w272 -> [w279 w287]
          frame "Dec", Default {
            n185 = call <userlib>:"Acm_AxStopDec.vi"("AxisHandle"=w279) -> ("ReturnValue"=w278:u32)  [unwired: 1 in, 2 out]
            n186 = Equal To 0?(x=w278) -> (x = 0?=w277:bool)
            n187 = Not(x=w277) -> (.not. x?=w276:bool)
            n188 = case shown="假" w276 {
              tunnel: w278 -> [_ w283]
              frame False {
              }
              frame True {
                n189 = Number To Hexadecimal String(2:w283) -> (0:w281:string)  [unwired: 1 out]
                n190 = Concatenate Strings("Stop failed with Error Code:0x", w281) -> (w280:string)
                n191 = One Button Dialog(message=w280) -> ()  [unwired: 2 out]
              }
            }
          }
          frame "Emg" {
            n192 = call <userlib>:"Acm_AxStopEmg.vi"("AxisHandle"=w287) -> ("ReturnValue"=w286:u32)  [unwired: 1 in, 2 out]
            n193 = Equal To 0?(x=w286) -> (x = 0?=w285:bool)
            n194 = Not(x=w285) -> (.not. x?=w284:bool)
            n195 = case shown="真" w284 {
              tunnel: w286 -> [_ w291]
              frame False {
              }
              frame True {
                n196 = Number To Hexadecimal String(2:w291) -> (0:w289:string)  [unwired: 1 out]
                n197 = Concatenate Strings("Stop failed with Error Code:0x", w289) -> (w288:string)
                n198 = One Button Dialog(message=w288) -> ()  [unwired: 2 out]
              }
            }
          }
        }
        n199 = local write "上行状态"(FALSE ("上行状态")) -> ()
        n200 = local write "上行停止状态"(FALSE ("上行停止状态")) -> ()
        n201 = local write "下行状态"(FALSE ("下行状态")) -> ()
        "下行停止状态" <- TRUE
      }
      frame "curve_return" {
        n202 = local write "automitic"(TRUE ("automitic")) -> ()
        n203 = local read "AxisHandle_Array"() -> (w295:u32[])
        n204 = Index Array(array=w295, index=4 ("索引")) -> (element=w296:u32)
        n205 = call <userlib>:"Acm_AxMoveVel.vi"("Direction"=u16 1, "AxisHandle"=w296) -> ()  [unwired: 1 in, 3 out]
        n206 = local write "下行状态"(FALSE ("下行状态")) -> ()
        n207 = local write "下行停止状态"(TRUE ("下行停止状态")) -> ()
        n208 = local write "上行状态"(TRUE ("上行状态")) -> ()
        n209 = local write "上行停止状态"(FALSE ("上行停止状态")) -> ()
      }
      frame "reset1" {
        w303 = 0.0 ("Position")
        n210 = local write "automitic"(TRUE ("automitic")) -> ()
        n211 = local read "AxisHandle_Array"() -> (w308:u32[])
        n212 = local write "运行状态"("Downward" ("运行状态")) -> ()
        n213 = Index Array(array=w308, index=4 ("索引")) -> (element=w306:u32)
        n214 = call <userlib>:"Acm_AxSetActualPosition.vi"("Position"=w303, "AxisHandle"=w306) -> ("ReturnValue"=w305:u32)  [unwired: 1 in, 2 out]
        n215 = local write "弯曲伺服"(w303) -> ()
        n216 = Equal To 0?(x=w305) -> (x = 0?=→"重置计数器成功":bool)
      }
      frame "stop1", Default {
        n217 = local write "automitic"(FALSE ("automitic")) -> ()
        n218 = local read "AxisHandle_Array"() -> (w316:u32[])
        n219 = Index Array(array=w316, index=4 ("索引")) -> (element=w312:u32)
        n220 = property on="停止1" class="Bool"("DisabledEnum"=T3."Disabled" ("禁用")) -> ()  [unwired: 2 in, 2 out]
        n221 = property on="弯曲" class="Bool"("DisabledEnum"=T3."Enabled" ("禁用")) -> ()  [unwired: 2 in, 2 out]
        n222 = case shown="\"Emg\"" "停止模式" {
          tunnel: w312 -> [w317 w328]
          frame "Dec", Default {
            n223 = call <userlib>:"Acm_AxStopDec.vi"("AxisHandle"=w317) -> ("ReturnValue"=w319:u32)  [unwired: 1 in, 2 out]
            n224 = Equal To 0?(x=w319) -> (x = 0?=w318:bool)
            "减速停止成功" <- w318
            n225 = Not(x=w318) -> (.not. x?=w320:bool)
            n226 = case shown="真" w320 {
              tunnel: w319 -> [_ w324]
              frame False {
              }
              frame True {
                n227 = Number To Hexadecimal String(2:w324) -> (0:w322:string)  [unwired: 1 out]
                n228 = Concatenate Strings("Stop Failed With Error Code:0x", w322) -> (w321:string)
                n229 = One Button Dialog(message=w321) -> ()  [unwired: 2 out]
              }
            }
          }
          frame "Emg" {
            n230 = call <userlib>:"Acm_AxStopEmg.vi"("AxisHandle"=w328) -> ("ReturnValue"=w327:u32)  [unwired: 1 in, 2 out]
            n231 = Equal To 0?(x=w327) -> (x = 0?=w325:bool)
            "急速停止成功" <- w325
            n232 = Not(x=w325) -> (.not. x?=w326:bool)
            n233 = case shown="真" w326 {
              tunnel: w327 -> [_ w332]
              frame False {
              }
              frame True {
                n234 = Number To Hexadecimal String(2:w332) -> (0:w330:string)  [unwired: 1 out]
                n235 = Concatenate Strings("Stop failed with Error Code:0x", w330) -> (w329:string)
                n236 = One Button Dialog(message=w329) -> ()  [unwired: 2 out]
              }
            }
          }
        }
      }
      frame "curve2" {
        n237 = local write "弯曲计算"("弯曲双线性" ("采集状态")) -> ()
      }
      frame "Reverse" {
        n238 = local write "automitic"(TRUE ("automitic")) -> ()
        n239 = local read "AxisHandle_Array"() -> (w347:u32[])
        n240 = local read "停止模式"() -> (w339:enum32{"Dec", "Emg"})
        n241 = property on="扭转" class="Bool"("DisabledEnum"=T3."Disabled" ("禁用")) -> ()  [unwired: 2 in, 2 out]
        n242 = property on="停止2" class="Bool"("DisabledEnum"=T3."Enabled" ("禁用")) -> ()  [unwired: 2 in, 2 out]
        n243 = Index Array(array=w347, index=5 ("索引")) -> (element=w338:u32)
        n244 = local write "拉伸停止"(FALSE ("拉伸停止")) -> ()
        n245 = disable-structure shown="启用" {
          disable-tunnel: "设定扭转距离" -> [w351 w496]
          disable-tunnel: "设置扭转速度" -> [w350 _]
          disable-tunnel: w339 -> [w349 _]
          disable-tunnel: w338 -> [w348 w495]
          frame Disabled {
            n246 = disable-structure shown="默认" {
              disable-tunnel: w351 -> [w356 _]
              disable-tunnel: w350 -> [w355 _]
              disable-tunnel: w349 -> [w354 _]
              disable-tunnel: w348 -> [w353 w431]
              frame Disabled {
                n247 = while {
                  tunnel: w353 -> [w363]
                  shift-right: [w361] -> _
                  shift-left: "start" -> [w362]
                  tunnel: w355 -> [w359]
                  tunnel: w356 -> [w358]
                  tunnel: w354 -> [w357]
                  stop <- w360 stop-if-true
                  n248 = case shown="\"start\"" w362 {
                    tunnel: w363 -> [w367 w392 w408 w417]
                    tunnel: w359 -> [_ w391 _ w420]
                    tunnel: w358 -> [_ w384 w405 w419]
                    tunnel: ["return" w390 w406 w415] -> w361
                    tunnel: [FALSE FALSE w403 FALSE] -> w360
                    tunnel: w357 -> [w364 _ _ _]
                    frame "stop", Default {
                      n249 = case shown="\"Dec\", 默认" w364 {
                        tunnel: w367 -> [w371 w379]
                        frame "Dec", Default {
                          n250 = call <userlib>:"Acm_AxStopDec.vi"("AxisHandle"=w371) -> ("ReturnValue"=w370:u32)  [unwired: 1 in, 2 out]
                          n251 = Equal To 0?(x=w370) -> (x = 0?=w369:bool)
                          n252 = Not(x=w369) -> (.not. x?=w368:bool)
                          n253 = case shown="假" w368 {
                            tunnel: w370 -> [_ w375]
                            frame False {
                            }
                            frame True {
                              n254 = Number To Hexadecimal String(2:w375) -> (0:w373:string)  [unwired: 1 out]
                              n255 = Concatenate Strings("Stop failed with Error Code:0x", w373) -> (w372:string)
                              n256 = One Button Dialog(message=w372) -> ()  [unwired: 2 out]
                            }
                          }
                        }
                        frame "Emg" {
                          n257 = call <userlib>:"Acm_AxStopEmg.vi"("AxisHandle"=w379) -> ("ReturnValue"=w378:u32)  [unwired: 1 in, 2 out]
                          n258 = Equal To 0?(x=w378) -> (x = 0?=w377:bool)
                          n259 = Not(x=w377) -> (.not. x?=w376:bool)
                          n260 = case shown="真" w376 {
                            tunnel: w378 -> [_ w383]
                            frame False {
                            }
                            frame True {
                              n261 = Number To Hexadecimal String(2:w383) -> (0:w381:string)  [unwired: 1 out]
                              n262 = Concatenate Strings("Stop failed with Error Code:0x", w381) -> (w380:string)
                              n263 = One Button Dialog(message=w380) -> ()  [unwired: 2 out]
                            }
                          }
                        }
                      }
                    }
                    frame "return" {
                      n264 = flat-sequence {
                        tunnel: w392 -> [w397]
                        tunnel: [w397] -> w394
                        tunnel: w394 -> [w399]
                        tunnel: [w399] -> w393
                        tunnel: w393 -> [w401]
                        tunnel: w391 -> [w402]
                        tunnel: [w401] -> w387
                        frame #0 {
                          n265 = call <userlib>:"Acm_AxSetSvOn.vi"("OnOff"=u32 1, "AxisHandle"=w397) -> ()  [unwired: 1 in, 3 out]
                        }
                        frame #1 {
                          n266 = call <userlib>:"Acm_AxMoveVel.vi"("Direction"=u16 1, "AxisHandle"=w399) -> ()  [unwired: 1 in, 3 out]
                        }
                        frame #2 {
                          n267 = call <userlib>:"Acm_AxChangeVel.vi"("NewVelocity"=w402, "AxisHandle"=w401) -> ()  [unwired: 1 in, 3 out]
                        }
                      }
                      n268 = call <userlib>:"Acm_AxGetCmdPosition.vi"("AxisHandle"=w387) -> ("Position"=w388:dbl)  [unwired: 1 in, 3 out]
                      n269 = Negate(x=w384) -> (-x=w385:dbl)
                      n270 = Less?(x=w388, y=w385) -> (x < y?=w386:bool)
                      n271 = case shown="假" w386 {
                        tunnel: ["return" "exit"] -> w390
                        frame False {
                        }
                        frame True {
                        }
                      }
                    }
                    frame "exit" {
                      n272 = call <userlib>:"Acm_AxGetCmdPosition.vi"("AxisHandle"=w408) -> ("Position"=w409:dbl)  [unwired: 1 in, 3 out]
                      n273 = Negate(x=w405) -> (-x=w404:dbl)
                      n274 = Equal?(x=w409, y=w404) -> (x = y?=w407:bool)
                      n275 = case shown="真" w407 {
                        tunnel: ["return" "exit"] -> w406
                        tunnel: [FALSE TRUE] -> w403
                        frame False {
                        }
                        frame True {
                        }
                      }
                    }
                    frame "start" {
                      n276 = flat-sequence {
                        tunnel: w417 -> [w425]
                        tunnel: [w425] -> w422
                        tunnel: w422 -> [w427]
                        tunnel: [w427] -> w421
                        tunnel: w421 -> [w430]
                        tunnel: w420 -> [w429]
                        frame #0 {
                          n277 = call <userlib>:"Acm_AxSetSvOn.vi"("OnOff"=u32 1, "AxisHandle"=w425) -> ()  [unwired: 1 in, 3 out]
                        }
                        frame #1 {
                          n278 = call <userlib>:"Acm_AxMoveVel.vi"("Direction"=u16 0, "AxisHandle"=w427) -> ()  [unwired: 1 in, 3 out]
                        }
                        frame #2 {
                          n279 = call <userlib>:"Acm_AxChangeVel.vi"("NewVelocity"=w429, "AxisHandle"=w430) -> ()  [unwired: 1 in, 3 out]
                        }
                      }
                      n280 = call <userlib>:"Acm_AxGetCmdPosition.vi"("AxisHandle"=w417) -> ("Position"=w418:dbl)  [unwired: 1 in, 3 out]
                      n281 = Greater?(x=w418, y=w419) -> (0:w416:bool)
                      n282 = case shown="真" w416 {
                        tunnel: ["start" "stop"] -> w415
                        frame False {
                        }
                        frame True {
                        }
                      }
                    }
                  }
                }
              }
              frame Enabled {
                n283 = disable-structure shown="默认" {
                  disable-tunnel: w431 -> [w432 w453]
                  frame Disabled {
                    n284 = stacked-sequence {
                      tunnel: w432 -> [w434 w436 w442 w443 w449 w452]
                      tunnel: [_ _ _ _ _ TRUE] -> _
                      frame #0 {
                        n285 = call <userlib>:"Acm_AxSetSvOn.vi"("OnOff"=u32 1, "AxisHandle"=w434) -> ()  [unwired: 1 in, 3 out]
                      }
                      frame #1 {
                        n286 = while {
                          tunnel: w436 -> [w439]
                          stop <- w440 stop-if-true
                          n287 = local read "设定扭转距离"() -> (w437:dbl)
                          n288 = call <userlib>:"Acm_AxGetActualPosition.vi"("AxisHandle"=w439) -> ("Position"=w438:dbl)  [unwired: 1 in, 3 out]
                          n289 = Greater?(x=w438, y=w437) -> (0:w440:bool)
                          n290 = local write "扭转伺服"(w438) -> ()
                        }
                        n291 = call <userlib>:"Acm_AxMoveVel.vi"("AxisHandle"=w436) -> ()  [unwired: 2 in, 3 out]
                      }
                      frame #2 {
                        n292 = call <userlib>:"Acm_AxStopEmg.vi"("AxisHandle"=w442) -> ()  [unwired: 1 in, 3 out]
                        n293 = Wait (ms)(milliseconds to wait=u32 2000 ("等待时间（毫秒）")) -> ()  [unwired: 1 out]
                      }
                      frame #3 {
                        n294 = while {
                          tunnel: w443 -> [w447]
                          stop <- w448 stop-if-true
                          n295 = call <userlib>:"Acm_AxGetActualPosition.vi"("AxisHandle"=w447) -> ("Position"=w445:dbl)  [unwired: 1 in, 3 out]
                          n296 = Less?(x=w445, y=20.0) -> (x < y?=w448:bool)
                          n297 = local write "扭转伺服"(w445) -> ()
                        }
                        n298 = call <userlib>:"Acm_AxMoveVel.vi"("Direction"=u16 1, "AxisHandle"=w443) -> ()  [unwired: 1 in, 3 out]
                      }
                      frame #4 {
                        n299 = call <userlib>:"Acm_AxStopEmg.vi"("AxisHandle"=w449) -> ()  [unwired: 1 in, 3 out]
                      }
                      frame #5 {
                        n300 = call <userlib>:"Acm_AxSetSvOn.vi"("OnOff"=u32 0, "AxisHandle"=w452) -> ()  [unwired: 1 in, 3 out]
                      }
                    }
                    n301 = call <userlib>:"Acm_AxSetActualPosition.vi"("Position"=0.0, "AxisHandle"=w432) -> ()  [unwired: 1 in, 3 out]
                  }
                  frame Enabled {
                    n302 = while {
                      tunnel: w453 -> [w462]
                      shift-right: [w459] -> _
                      shift-left: "server_on" -> [w461]
                      stop <- w460 stop-if-true
                      n303 = local read "设定扭转距离"() -> (w456:dbl)
                      n304 = call <userlib>:"Acm_AxGetActualPosition.vi"("AxisHandle"=w462) -> ("Position"=w457:dbl)  [unwired: 1 in, 3 out]
                      n305 = Greater?(x=w457, y=w456) -> (0:w458:bool)
                      n306 = case shown="\"server_off\"" w461 {
                        tunnel: w462 -> [w465 w471 w476 w483 w489 w492]
                        tunnel: w457 -> [_ _ _ w482 _ _]
                        tunnel: [FALSE FALSE FALSE FALSE FALSE TRUE] -> w460
                        tunnel: ["positive" w467 "Reverse" w479 "server_off" "server_off"] -> w459
                        tunnel: w458 -> [_ w469 _ _ _ _]
                        frame "server_on" {
                          n307 = call <userlib>:"Acm_AxSetSvOn.vi"("OnOff"=u32 1, "AxisHandle"=w465) -> ()  [unwired: 1 in, 3 out]
                        }
                        frame "positive", Default {
                          n308 = call <userlib>:"Acm_AxMoveVel.vi"("Direction"=u16 0, "AxisHandle"=w471) -> ()  [unwired: 1 in, 3 out]
                          n309 = case shown="真" w469 {
                            tunnel: ["positive" "stop1"] -> w467
                            frame False {
                            }
                            frame True {
                            }
                          }
                        }
                        frame "stop1" {
                          n310 = call <userlib>:"Acm_AxStopEmg.vi"("AxisHandle"=w476) -> ()  [unwired: 1 in, 3 out]
                          n311 = Wait (ms)(milliseconds to wait=u32 2000 ("等待时间（毫秒）")) -> ()  [unwired: 1 out]
                        }
                        frame "Reverse" {
                          n312 = call <userlib>:"Acm_AxMoveVel.vi"("Direction"=u16 1, "AxisHandle"=w483) -> ()  [unwired: 1 in, 3 out]
                          n313 = Less?(x=w482, y=20.0) -> (x < y?=w480:bool)
                          n314 = case shown="真" w480 {
                            tunnel: ["Reverse" "stop"] -> w479
                            frame False {
                            }
                            frame True {
                            }
                          }
                        }
                        frame "stop" {
                          n315 = call <userlib>:"Acm_AxStopEmg.vi"("AxisHandle"=w489) -> ()  [unwired: 1 in, 3 out]
                        }
                        frame "server_off" {
                          n316 = call <userlib>:"Acm_AxSetSvOn.vi"("OnOff"=u32 0, "AxisHandle"=w492) -> ()  [unwired: 1 in, 3 out]
                        }
                      }
                      n317 = local write "扭转伺服"(w457) -> ()
                    }
                    n318 = call <userlib>:"Acm_AxSetActualPosition.vi"("Position"=0.0, "AxisHandle"=w453) -> ()  [unwired: 1 in, 3 out]
                  }
                }
              }
            }
          }
          frame Enabled {
            n319 = case shown="\"Downward\", 默认" "运行状态 2" {
              tunnel: w495 -> [w502 w516 w529]
              tunnel: w496 -> [w503 w515 w528]
              frame "Downward", Default {
                n320 = flat-sequence {
                  tunnel: w502 -> [w504]
                  tunnel: w502 -> [w507]
                  tunnel: w502 -> [w509]
                  tunnel: w503 -> [w508]
                  frame #0 {
                    n321 = call <userlib>:"Acm_AxSetSvOn.vi"("OnOff"=u32 1, "AxisHandle"=w504) -> ()  [unwired: 1 in, 3 out]
                  }
                  frame #1 {
                    n322 = call <userlib>:"Acm_AxMoveVel.vi"("Direction"=u16 0, "AxisHandle"=w507) -> ()  [unwired: 1 in, 3 out]
                  }
                  frame #2 {
                    n323 = call <userlib>:"Acm_AxChangeVel.vi"("NewVelocity"=w508, "AxisHandle"=w509) -> ()  [unwired: 1 in, 3 out]
                  }
                }
                n324 = local write "下行停止状态 2"(FALSE ("下行停止状态")) -> ()
                n325 = local write "下行状态 2"(TRUE ("下行状态")) -> ()
                n326 = local write "上行状态 2"(FALSE ("上行状态")) -> ()
                n327 = local write "上行停止状态 2"(FALSE ("上行停止状态")) -> ()
                n328 = local write "运行状态 2"("Downward" ("运行状态")) -> ()
              }
              frame "Up-going" {
                n329 = flat-sequence {
                  tunnel: w516 -> [w517]
                  tunnel: w516 -> [w519]
                  tunnel: w516 -> [w522]
                  tunnel: w515 -> [w521]
                  frame #0 {
                    n330 = call <userlib>:"Acm_AxSetSvOn.vi"("OnOff"=u32 1, "AxisHandle"=w517) -> ()  [unwired: 1 in, 3 out]
                  }
                  frame #1 {
                    n331 = call <userlib>:"Acm_AxMoveVel.vi"("Direction"=u16 1, "AxisHandle"=w519) -> ()  [unwired: 1 in, 3 out]
                  }
                  frame #2 {
                    n332 = call <userlib>:"Acm_AxChangeVel.vi"("NewVelocity"=w521, "AxisHandle"=w522) -> ()  [unwired: 1 in, 3 out]
                  }
                }
                n333 = local write "下行停止状态 2"(FALSE ("下行停止状态")) -> ()
                n334 = local write "下行状态 2"(FALSE ("下行状态")) -> ()
                n335 = local write "上行停止状态 2"(TRUE ("上行停止状态")) -> ()
                n336 = local write "上行状态 2"(TRUE ("上行状态")) -> ()
                n337 = local write "运行状态 2"("Up-going" ("运行状态")) -> ()
              }
              frame "initialization" {
                n338 = flat-sequence {
                  tunnel: w529 -> [w530]
                  tunnel: w529 -> [w532]
                  tunnel: w529 -> [w535]
                  tunnel: w528 -> [w534]
                  frame #0 {
                    n339 = call <userlib>:"Acm_AxSetSvOn.vi"("OnOff"=u32 1, "AxisHandle"=w530) -> ()  [unwired: 1 in, 3 out]
                  }
                  frame #1 {
                    n340 = call <userlib>:"Acm_AxMoveVel.vi"("Direction"=u16 0, "AxisHandle"=w532) -> ()  [unwired: 1 in, 3 out]
                  }
                  frame #2 {
                    n341 = call <userlib>:"Acm_AxChangeVel.vi"("NewVelocity"=w534, "AxisHandle"=w535) -> ()  [unwired: 1 in, 3 out]
                  }
                }
                n342 = local write "运行状态 2"("Downward" ("运行状态")) -> ()
                "下行停止状态 2" <- FALSE ("下行停止状态")
                "上行状态 2" <- FALSE ("上行状态")
                "上行停止状态 2" <- FALSE ("上行停止状态")
                "下行状态 2" <- TRUE ("下行状态")
              }
            }
          }
        }
        n343 = call <userlib>:"Acm_AxGetActualPosition.vi"("AxisHandle"=w338) -> ("ReturnValue"=w343:u32, "AxisHandle"=w344:u32)  [unwired: 1 in, 2 out]
        n344 = call <userlib>:"Acm_AxGetActVelocity.vi"("AxisHandle"=w338) -> ("Velocity"=→"当前指令的速度 2":dbl)  [unwired: 1 in, 3 out]
        n345 = Equal To 0?(x=w343) -> (x = 0?=w342:bool)
        n346 = case shown="真" w342 {
          tunnel: w344 -> [_ w536]
          frame False {
          }
          frame True {
            n347 = case shown="0, 默认" w536 {
              frame 0, Default {
                "轴的状态: 2" <- "Axis is disabled." ("Axis State:")
              }
              frame 1 {
                n348 = local write "轴的状态: 2"("Axis is ready." ("Axis State:")) -> ()
              }
              frame 2 {
                n349 = local write "轴的状态: 2"("Axis is stopping." ("Axis State:")) -> ()
              }
              frame 3 {
                n350 = local write "轴的状态: 2"("Axis is Error_Stopped." ("Axis State:")) -> ()
              }
              frame 4 {
                n351 = local write "轴的状态: 2"("Axis is executing home motion." ("Axis State:")) -> ()
              }
              frame 5 {
                n352 = local write "轴的状态: 2"("Axis is executing PTP motion." ("Axis State:")) -> ()
              }
              frame 6 {
                n353 = local write "轴的状态: 2"("Axis is executing continuous motion." ("Axis State:")) -> ()
              }
              frame 7 {
                n354 = local write "轴的状态: 2"("Axis is in Group interpolation motion." ("Axis State:")) -> ()
              }
              frame 8 {
                n355 = local write "轴的状态: 2"("Axis is executing JOG mode motion." ("Axis State:")) -> ()
              }
              frame 9 {
                n356 = local write "轴的状态: 2"("Axis is executing MPG mode motion." ("Axis State:")) -> ()
              }
            }
          }
        }
      }
      frame "Reverse_stop" {
        n357 = local write "automitic"(TRUE ("automitic")) -> ()
        n358 = local read "AxisHandle_Array"() -> (w555:u32[])
        n359 = local write "下行停止状态 2"(TRUE ("下行停止状态")) -> ()
        n360 = local write "下行状态 2"(FALSE ("下行状态")) -> ()
        n361 = Index Array(array=w555, index=5 ("索引")) -> (element=w552:u32)
        n362 = local write "上行状态 2"(FALSE ("上行状态")) -> ()
        n363 = local write "上行停止状态 2"(FALSE ("上行停止状态")) -> ()
        n364 = local read "停止模式"() -> (w553:enum32{"Dec", "Emg"})
        n365 = case shown="\"Emg\"" w553 {
          tunnel: w552 -> [w559 w567]
          frame "Dec", Default {
            n366 = call <userlib>:"Acm_AxStopDec.vi"("AxisHandle"=w559) -> ("ReturnValue"=w558:u32)  [unwired: 1 in, 2 out]
            n367 = Equal To 0?(x=w558) -> (x = 0?=w557:bool)
            n368 = Not(x=w557) -> (.not. x?=w556:bool)
            n369 = case shown="真" w556 {
              tunnel: w558 -> [_ w563]
              frame False {
              }
              frame True {
                n370 = Number To Hexadecimal String(2:w563) -> (0:w561:string)  [unwired: 1 out]
                n371 = Concatenate Strings("Stop failed with Error Code:0x", w561) -> (w560:string)
                n372 = One Button Dialog(message=w560) -> ()  [unwired: 2 out]
              }
            }
          }
          frame "Emg" {
            n373 = call <userlib>:"Acm_AxStopEmg.vi"("AxisHandle"=w567) -> ("ReturnValue"=w566:u32)  [unwired: 1 in, 2 out]
            n374 = Equal To 0?(x=w566) -> (x = 0?=w565:bool)
            n375 = Not(x=w565) -> (.not. x?=w564:bool)
            n376 = case shown="真" w564 {
              tunnel: w566 -> [_ w571]
              frame False {
              }
              frame True {
                n377 = Number To Hexadecimal String(2:w571) -> (0:w569:string)  [unwired: 1 out]
                n378 = Concatenate Strings("Stop failed with Error Code:0x", w569) -> (w568:string)
                n379 = One Button Dialog(message=w568) -> ()  [unwired: 2 out]
              }
            }
          }
        }
      }
      frame "reverse_return" {
        n380 = local write "automitic"(TRUE ("automitic")) -> ()
        n381 = local read "AxisHandle_Array"() -> (w581:u32[])
        n382 = Index Array(array=w581, index=5 ("索引")) -> (element=w579:u32)
        n383 = call <userlib>:"Acm_AxMoveVel.vi"("Direction"=u16 1, "AxisHandle"=w579) -> ()  [unwired: 1 in, 3 out]
        n384 = local write "拉伸停止"(FALSE ("拉伸停止")) -> ()
        n385 = local write "下行停止状态 2"(TRUE ("下行停止状态")) -> ()
        n386 = local write "下行状态 2"(FALSE ("下行状态")) -> ()
        n387 = local write "上行状态 2"(TRUE ("上行状态")) -> ()
        n388 = local write "上行停止状态 2"(FALSE ("上行停止状态")) -> ()
      }
      frame "reset2" {
        n389 = local write "automitic"(FALSE ("automitic")) -> ()
        n390 = local read "轴打开成功"() -> (w583:bool)
        n391 = case shown="真" w583 {
          frame False {
          }
          frame True {
            w585 = 0.0 ("Position")
            n392 = local read "AxisHandle_Array"() -> (w590:u32[])
            n393 = local write "运行状态 2"("Downward" ("运行状态 2")) -> ()
            n394 = Index Array(array=w590, index=5 ("索引")) -> (element=w589:u32)
            n395 = call <userlib>:"Acm_AxSetActualPosition.vi"("Position"=w585, "AxisHandle"=w589) -> ("ReturnValue"=w588:u32)  [unwired: 1 in, 2 out]
            n396 = Equal To 0?(x=w588) -> (x = 0?=→"重置计数器成功 2":bool)
            "扭转伺服" <- w585
          }
        }
      }
      frame "stop2" {
        n397 = local write "automitic"(FALSE ("automitic")) -> ()
        n398 = local read "AxisHandle_Array"() -> (w597:u32[])
        n399 = Index Array(array=w597, index=5 ("索引")) -> (element=w594:u32)
        n400 = local read "停止模式"() -> (w595:enum32{"Dec", "Emg"})
        n401 = property on="扭转" class="Bool"("DisabledEnum"=T3."Enabled" ("禁用")) -> ()  [unwired: 2 in, 2 out]
        n402 = property on="停止2" class="Bool"("DisabledEnum"=T3."Disabled" ("禁用")) -> ()  [unwired: 2 in, 2 out]
        n403 = case shown="\"Emg\"" w595 {
          tunnel: w594 -> [w601 w609]
          frame "Dec", Default {
            n404 = call <userlib>:"Acm_AxStopDec.vi"("AxisHandle"=w601) -> ("ReturnValue"=w600:u32)  [unwired: 1 in, 2 out]
            n405 = Equal To 0?(x=w600) -> (x = 0?=w599:bool)
            n406 = Not(x=w599) -> (.not. x?=w598:bool)
            n407 = case shown="真" w598 {
              tunnel: w600 -> [_ w605]
              frame False {
              }
              frame True {
                n408 = Number To Hexadecimal String(2:w605) -> (0:w603:string)  [unwired: 1 out]
                n409 = Concatenate Strings("Stop failed with Error Code:0x", w603) -> (w602:string)
                n410 = One Button Dialog(message=w602) -> ()  [unwired: 2 out]
              }
            }
          }
          frame "Emg" {
            n411 = call <userlib>:"Acm_AxStopEmg.vi"("AxisHandle"=w609) -> ("ReturnValue"=w608:u32)  [unwired: 1 in, 2 out]
            n412 = Equal To 0?(x=w608) -> (x = 0?=w607:bool)
            n413 = Not(x=w607) -> (.not. x?=w606:bool)
            n414 = case shown="真" w606 {
              tunnel: w608 -> [_ w613]
              frame False {
              }
              frame True {
                n415 = Number To Hexadecimal String(2:w613) -> (0:w611:string)  [unwired: 1 out]
                n416 = Concatenate Strings("Stop failed with Error Code:0x", w611) -> (w610:string)
                n417 = One Button Dialog(message=w610) -> ()  [unwired: 2 out]
              }
            }
          }
        }
      }
      frame "Stretch" {
        n418 = local write "automitic"(TRUE ("automitic")) -> ()
        n419 = local read "AxisHandle_Array"() -> (w628:u32[])
        n420 = Index Array(array=w628, index=6 ("索引")) -> (element=w619:u32)
        n421 = property on="手动" class="Bool"("DisabledEnum"=T3."Disabled" ("禁用")) -> ()  [unwired: 2 in, 2 out]
        n422 = property on="停止3" class="Bool"("DisabledEnum"=T3."Enabled" ("禁用")) -> ()  [unwired: 2 in, 2 out]
        n423 = property on="拉伸" class="Bool"("DisabledEnum"=T3."Disabled" ("禁用")) -> ()  [unwired: 2 in, 2 out]
        n424 = call <userlib>:"Acm_AxGetState.vi"("AxisHandle"=w619) -> ("ReturnValue"=w625:u32, "Status"=w626:u16)  [unwired: 1 in, 2 out]
        n425 = call <userlib>:"Acm_AxGetCmdVelocity.vi"("AxisHandle"=w619) -> ("Velocity"=→"当前指令的速度 3":dbl)  [unwired: 1 in, 3 out]
        n426 = case shown="\"Downward\", 默认" "运行状态 3" {
          tunnel: w619 -> [w635 w650 w664]
          tunnel: "设置拉伸速度" -> [w636 w649 w663]
          frame "Downward", Default {
            n427 = local write "拉伸停止"(FALSE ("拉伸停止")) -> ()
            n428 = flat-sequence {
              tunnel: w635 -> [w637]
              tunnel: w635 -> [w640]
              tunnel: w635 -> [w642]
              tunnel: w636 -> [w641]
              frame #0 {
                n429 = call <userlib>:"Acm_AxSetSvOn.vi"("OnOff"=u32 1, "AxisHandle"=w637) -> ()  [unwired: 1 in, 3 out]
              }
              frame #1 {
                n430 = call <userlib>:"Acm_AxMoveVel.vi"("Direction"=u16 0, "AxisHandle"=w640) -> ()  [unwired: 1 in, 3 out]
              }
              frame #2 {
                n431 = call <userlib>:"Acm_AxChangeVel.vi"("NewVelocity"=w641, "AxisHandle"=w642) -> ()  [unwired: 1 in, 3 out]
              }
            }
            n432 = local write "运行状态 3"("Downward" ("运行状态")) -> ()
            "下行停止状态 3" <- FALSE ("下行停止状态")
            "上行状态 3" <- FALSE ("上行状态")
            "下行状态 3" <- TRUE ("下行状态")
            "上行停止状态 3" <- FALSE ("上行停止状态")
          }
          frame "Up-going" {
            n433 = flat-sequence {
              tunnel: w650 -> [w651]
              tunnel: w650 -> [w653]
              tunnel: w650 -> [w656]
              tunnel: w649 -> [w655]
              frame #0 {
                n434 = call <userlib>:"Acm_AxSetSvOn.vi"("OnOff"=u32 1, "AxisHandle"=w651) -> ()  [unwired: 1 in, 3 out]
              }
              frame #1 {
                n435 = call <userlib>:"Acm_AxMoveVel.vi"("Direction"=u16 1, "AxisHandle"=w653) -> ()  [unwired: 1 in, 3 out]
              }
              frame #2 {
                n436 = call <userlib>:"Acm_AxChangeVel.vi"("NewVelocity"=w655, "AxisHandle"=w656) -> ()  [unwired: 1 in, 3 out]
              }
            }
            n437 = local write "下行停止状态 3"(FALSE ("下行停止状态")) -> ()
            n438 = local write "下行状态 3"(FALSE ("下行状态")) -> ()
            n439 = local write "拉伸停止"(FALSE ("拉伸停止")) -> ()
            n440 = local write "上行停止状态 3"(TRUE ("上行停止状态")) -> ()
            n441 = local write "上行状态 3"(TRUE ("上行状态")) -> ()
            n442 = local write "运行状态 3"("Up-going" ("运行状态")) -> ()
          }
          frame "initialization" {
            n443 = local write "拉伸停止"(FALSE ("拉伸停止")) -> ()
            n444 = local write "下行停止状态 3"(FALSE ("下行停止状态")) -> ()
            n445 = local write "下行状态 3"(TRUE ("下行状态")) -> ()
            n446 = flat-sequence {
              tunnel: w664 -> [w665]
              tunnel: w664 -> [w667]
              tunnel: w664 -> [w670]
              tunnel: w663 -> [w669]
              frame #0 {
                n447 = call <userlib>:"Acm_AxSetSvOn.vi"("OnOff"=u32 1, "AxisHandle"=w665) -> ()  [unwired: 1 in, 3 out]
              }
              frame #1 {
                n448 = call <userlib>:"Acm_AxMoveVel.vi"("Direction"=u16 0, "AxisHandle"=w667) -> ()  [unwired: 1 in, 3 out]
              }
              frame #2 {
                n449 = call <userlib>:"Acm_AxChangeVel.vi"("NewVelocity"=w669, "AxisHandle"=w670) -> ()  [unwired: 1 in, 3 out]
              }
            }
            n450 = local write "上行停止状态 3"(FALSE ("上行停止状态")) -> ()
            n451 = local write "上行状态 3"(FALSE ("上行状态")) -> ()
            n452 = local write "运行状态 3"("Downward" ("运行状态")) -> ()
          }
        }
        n453 = Equal To 0?(x=w625) -> (x = 0?=w624:bool)
        n454 = case shown="真" w624 {
          tunnel: w626 -> [_ w671]
          frame False {
          }
          frame True {
            n455 = case shown="1" w671 {
              frame 0, Default {
                n456 = local write "轴的状态: 3"("Axis is disabled." ("Axis State:")) -> ()
              }
              frame 1 {
                "轴的状态: 3" <- "Axis is ready." ("Axis State:")
              }
              frame 2 {
                n457 = local write "轴的状态: 3"("Axis is stopping." ("Axis State:")) -> ()
              }
              frame 3 {
                n458 = local write "轴的状态: 3"("Axis is Error_Stopped." ("Axis State:")) -> ()
              }
              frame 4 {
                n459 = local write "轴的状态: 3"("Axis is executing home motion." ("Axis State:")) -> ()
              }
              frame 5 {
                n460 = local write "轴的状态: 3"("Axis is executing PTP motion." ("Axis State:")) -> ()
              }
              frame 6 {
                n461 = local write "轴的状态: 3"("Axis is executing continuous motion." ("Axis State:")) -> ()
              }
              frame 7 {
                n462 = local write "轴的状态: 3"("Axis is in Group interpolation motion." ("Axis State:")) -> ()
              }
              frame 8 {
                n463 = local write "轴的状态: 3"("Axis is executing JOG mode motion." ("Axis State:")) -> ()
              }
              frame 9 {
                n464 = local write "轴的状态: 3"("Axis is executing MPG mode motion." ("Axis State:")) -> ()
              }
            }
          }
        }
        "当前温度" <- "设定温度"
        "当前压力" <- "设定压力"
      }
      frame "Stretch_stop" {
        n465 = local write "automitic"(TRUE ("automitic")) -> ()
        n466 = local read "AxisHandle_Array"() -> (w686:u32[])
        n467 = local read "停止模式"() -> (w684:enum32{"Dec", "Emg"})
        n468 = local write "下行停止状态 3"(TRUE ("下行停止状态")) -> ()
        n469 = local write "下行状态 3"(FALSE ("下行状态")) -> ()
        n470 = Index Array(array=w686, index=6 ("索引")) -> (element=w683:u32)
        n471 = local write "上行停止状态 3"(FALSE ("上行停止状态")) -> ()
        n472 = local write "上行状态 3"(FALSE ("上行状态")) -> ()
        n473 = case shown="\"Dec\", 默认" w684 {
          tunnel: w683 -> [w694 w702]
          frame "Dec", Default {
            n474 = call <userlib>:"Acm_AxStopDec.vi"("AxisHandle"=w694) -> ("ReturnValue"=w693:u32)  [unwired: 1 in, 2 out]
            n475 = Equal To 0?(x=w693) -> (x = 0?=w692:bool)
            n476 = Not(x=w692) -> (.not. x?=w691:bool)
            n477 = case shown="真" w691 {
              tunnel: w693 -> [_ w698]
              frame False {
              }
              frame True {
                n478 = Number To Hexadecimal String(2:w698) -> (0:w696:string)  [unwired: 1 out]
                n479 = Concatenate Strings("Stop failed with Error Code:0x", w696) -> (w695:string)
                n480 = One Button Dialog(message=w695) -> ()  [unwired: 2 out]
              }
            }
          }
          frame "Emg" {
            n481 = call <userlib>:"Acm_AxStopEmg.vi"("AxisHandle"=w702) -> ("ReturnValue"=w701:u32)  [unwired: 1 in, 2 out]
            n482 = Equal To 0?(x=w701) -> (x = 0?=w700:bool)
            n483 = Not(x=w700) -> (.not. x?=w699:bool)
            n484 = case shown="真" w699 {
              tunnel: w701 -> [_ w706]
              frame False {
              }
              frame True {
                n485 = Number To Hexadecimal String(2:w706) -> (0:w704:string)  [unwired: 1 out]
                n486 = Concatenate Strings("Stop failed with Error Code:0x", w704) -> (w703:string)
                n487 = One Button Dialog(message=w703) -> ()  [unwired: 2 out]
              }
            }
          }
        }
      }
      frame "Stretch_return" {
        n488 = local write "automitic"(TRUE ("automitic")) -> ()
        n489 = local read "AxisHandle_Array"() -> (w716:u32[])
        n490 = local write "下行停止状态 3"(TRUE ("下行停止状态")) -> ()
        n491 = local write "下行状态 3"(FALSE ("下行状态")) -> ()
        n492 = Index Array(array=w716, index=6 ("索引")) -> (element=w714:u32)
        n493 = call <userlib>:"Acm_AxMoveVel.vi"("Direction"=u16 1, "AxisHandle"=w714) -> ()  [unwired: 1 in, 3 out]
        n494 = local write "上行停止状态 3"(FALSE ("上行停止状态")) -> ()
        n495 = local write "上行状态 3"(TRUE ("上行状态")) -> ()
        n496 = local write "拉伸停止"(FALSE ("拉伸停止")) -> ()
      }
      frame "reset3" {
        n497 = local write "automitic"(TRUE ("automitic")) -> ()
        n498 = local read "轴打开成功"() -> (w719:bool)
        n499 = case shown="真" w719 {
          frame False {
          }
          frame True {
            w722 = 0.0 ("Position")
            n500 = local read "AxisHandle_Array"() -> (w726:u32[])
            n501 = local write "运行状态 3"("Downward" ("运行状态 3")) -> ()
            n502 = Index Array(array=w726, index=6 ("索引")) -> (element=w725:u32)
            n503 = call <userlib>:"Acm_AxSetActualPosition.vi"("Position"=w722, "AxisHandle"=w725) -> ("ReturnValue"=w724:u32)  [unwired: 1 in, 2 out]
            n504 = Equal To 0?(x=w724) -> (x = 0?=→"重置计数器成功 3":bool)
            "拉伸伺服" <- w722
          }
        }
        n505 = local write "拉伸停止"(FALSE ("拉伸停止")) -> ()
      }
      frame "stop3" {
        n506 = local write "automitic"(TRUE ("automitic")) -> ()
        n507 = local read "AxisHandle_Array"() -> (w733:u32[])
        n508 = Index Array(array=w733, index=6 ("索引")) -> (element=w730:u32)
        n509 = property on="停止3" class="Bool"("DisabledEnum"=T3."Disabled" ("禁用")) -> ()  [unwired: 2 in, 2 out]
        n510 = property on="拉伸" class="Bool"("DisabledEnum"=T3."Enabled" ("禁用")) -> ()  [unwired: 2 in, 2 out]
        n511 = local read "停止模式"() -> (w731:enum32{"Dec", "Emg"})
        n512 = disable-structure shown="禁用" {
          disable-tunnel: w730 -> [w750 _]
          frame Disabled {
            n513 = call <userlib>:"Acm_AxSetSvOn.vi"("OnOff"=u32 0, "AxisHandle"=w750) -> ("ReturnValue"=w753:u32)  [unwired: 1 in, 2 out]
            n514 = Not Equal To 0?(x=w753) -> (x != 0?=w752:bool)
            n515 = case shown="真" w752 {
              tunnel: w753 -> [_ w754]
              frame False {
              }
              frame True {
                w757 = "Servo On/Off Failed With Error Code:0x"  # Servo On/Off Failed With Error Code:0x
                n516 = Number To Hexadecimal String(2:w754) -> (0:w756:string)  [unwired: 1 out]
                n517 = Concatenate Strings(w757, w756) -> (w755:string)
                n518 = One Button Dialog(message=w755) -> ()  [unwired: 2 out]
              }
            }
          }
          frame Enabled {
          }
        }
        n519 = case shown="\"Dec\", 默认" w731 {
          tunnel: w730 -> [w737 w745]
          frame "Dec", Default {
            n520 = call <userlib>:"Acm_AxStopDec.vi"("AxisHandle"=w737) -> ("ReturnValue"=w736:u32)  [unwired: 1 in, 2 out]
            n521 = Equal To 0?(x=w736) -> (x = 0?=w735:bool)
            n522 = Not(x=w735) -> (.not. x?=w734:bool)
            n523 = case shown="真" w734 {
              tunnel: w736 -> [_ w741]
              frame False {
              }
              frame True {
                n524 = Number To Hexadecimal String(2:w741) -> (0:w739:string)  [unwired: 1 out]
                n525 = Concatenate Strings("Stop failed with Error Code:0x", w739) -> (w738:string)
                n526 = One Button Dialog(message=w738) -> ()  [unwired: 2 out]
              }
            }
          }
          frame "Emg" {
            n527 = call <userlib>:"Acm_AxStopEmg.vi"("AxisHandle"=w745) -> ("ReturnValue"=w744:u32)  [unwired: 1 in, 2 out]
            n528 = Equal To 0?(x=w744) -> (x = 0?=w743:bool)
            n529 = Not(x=w743) -> (.not. x?=w742:bool)
            n530 = case shown="真" w742 {
              tunnel: w744 -> [_ w749]
              frame False {
              }
              frame True {
                n531 = Number To Hexadecimal String(2:w749) -> (0:w747:string)  [unwired: 1 out]
                n532 = Concatenate Strings("Stop failed with Error Code:0x", w747) -> (w746:string)
                n533 = One Button Dialog(message=w746) -> ()  [unwired: 2 out]
              }
            }
          }
        }
      }
      frame "automatic" {
        n534 = local write "automitic"(TRUE ("automitic")) -> ()
      }
      frame "manual control" {
        n535 = local write "automitic"(FALSE ("automitic")) -> ()
        n536 = local read "AxisHandle_Array"() -> (w765:u32[])
        n537 = flat-sequence {
          tunnel: w763 -> [w766]
          tunnel: w763 -> [w774]
          frame #0 {
            n538 = call <userlib>:"Acm_AxSetSvOn.vi"("OnOff"=u32 1, "AxisHandle"=w766) -> ("ReturnValue"=w767:u32)  [unwired: 1 in, 2 out]
            n539 = Not Equal To 0?(x=w767) -> (x != 0?=w768:bool)
            n540 = case shown="真" w768 {
              tunnel: w767 -> [_ w770]
              frame False {
              }
              frame True {
                w773 = "Servo On/Off Failed With Error Code:0x"  # Servo On/Off Failed With Error Code:0x
                n541 = Number To Hexadecimal String(2:w770) -> (0:w772:string)  [unwired: 1 out]
                n542 = Concatenate Strings(w773, w772) -> (w771:string)
                n543 = One Button Dialog(message=w771) -> ()  [unwired: 2 out]
              }
            }
          }
          frame #1 {
            n544 = case shown="假" "手动方向" {
              tunnel: [enum32{"Negative", "Positive"}."Positive" ("Direction 2") enum32{"Negative", "Positive"}."Negative" ("Direction 2")] -> w775
              frame False {
              }
              frame True {
              }
            }
            n545 = case shown="\"Positive\"" w775 {
              tunnel: w774 -> [w780 w782]
              frame "Negative", Default {
                n546 = call <userlib>:"Acm_AxMoveVel.vi"("Direction"=u16 1, "AxisHandle"=w780) -> ()  [unwired: 1 in, 3 out]
              }
              frame "Positive" {
                n547 = call <userlib>:"Acm_AxMoveVel.vi"("Direction"=u16 0, "AxisHandle"=w782) -> ()  [unwired: 1 in, 3 out]
              }
            }
          }
        }
        n548 = Index Array(array=w765, index=6 ("索引")) -> (element=w763:u32)
        n549 = property on="手动" class="Bool"("DisabledEnum"=T3."Enabled" ("禁用")) -> ()  [unwired: 2 in, 2 out]
        n550 = property on="停止3" class="Bool"("DisabledEnum"=T3."Disabled" ("禁用")) -> ()  [unwired: 2 in, 2 out]
        n551 = property on="拉伸" class="Bool"("DisabledEnum"=T3."Disabled" ("禁用")) -> ()  [unwired: 2 in, 2 out]
      }
      frame "stop3_leave" {
        n552 = local read "AxisHandle_Array"() -> (w788:u32[])
        n553 = property on="手动" class="Bool"("DisabledEnum"=T3."Enabled" ("禁用")) -> ()  [unwired: 2 in, 2 out]
        n554 = property on="停止3" class="Bool"("DisabledEnum"=T3."Enabled" ("禁用")) -> ()  [unwired: 2 in, 2 out]
        n555 = property on="拉伸" class="Bool"("DisabledEnum"=T3."Enabled" ("禁用")) -> ()  [unwired: 2 in, 2 out]
        n556 = Index Array(array=w788, index=6 ("索引")) -> (element=w786:u32)
        n557 = stacked-sequence {
          tunnel: w786 -> [w791 w797]
          frame #0 {
            n558 = call <userlib>:"Acm_AxSetSvOn.vi"("OnOff"=u32 0, "AxisHandle"=w791) -> ("ReturnValue"=w789:u32)  [unwired: 1 in, 2 out]
            n559 = Not Equal To 0?(x=w789) -> (x != 0?=w790:bool)
            n560 = case shown="真" w790 {
              tunnel: w789 -> [_ w793]
              frame False {
              }
              frame True {
                w796 = "Servo On/Off Failed With Error Code:0x"  # Servo On/Off Failed With Error Code:0x
                n561 = Number To Hexadecimal String(2:w793) -> (0:w795:string)  [unwired: 1 out]
                n562 = Concatenate Strings(w796, w795) -> (w794:string)
                n563 = One Button Dialog(message=w794) -> ()  [unwired: 2 out]
              }
            }
          }
          frame #1 {
            n564 = local read "停止模式"() -> (w798:enum32{"Dec", "Emg"})
            n565 = case shown="\"Dec\", 默认" w798 {
              tunnel: w797 -> [w802 w810]
              frame "Dec", Default {
                n566 = call <userlib>:"Acm_AxStopDec.vi"("AxisHandle"=w802) -> ("ReturnValue"=w801:u32)  [unwired: 1 in, 2 out]
                n567 = Equal To 0?(x=w801) -> (x = 0?=w800:bool)
                n568 = Not(x=w800) -> (.not. x?=w799:bool)
                n569 = case shown="真" w799 {
                  tunnel: w801 -> [_ w806]
                  frame False {
                  }
                  frame True {
                    n570 = Number To Hexadecimal String(2:w806) -> (0:w804:string)  [unwired: 1 out]
                    n571 = Concatenate Strings("Stop failed with Error Code:0x", w804) -> (w803:string)
                    n572 = One Button Dialog(message=w803) -> ()  [unwired: 2 out]
                  }
                }
              }
              frame "Emg" {
                n573 = call <userlib>:"Acm_AxStopEmg.vi"("AxisHandle"=w810) -> ("ReturnValue"=w809:u32)  [unwired: 1 in, 2 out]
                n574 = Equal To 0?(x=w809) -> (x = 0?=w808:bool)
                n575 = Not(x=w808) -> (.not. x?=w807:bool)
                n576 = case shown="真" w807 {
                  tunnel: w809 -> [_ w814]
                  frame False {
                  }
                  frame True {
                    n577 = Number To Hexadecimal String(2:w814) -> (0:w812:string)  [unwired: 1 out]
                    n578 = Concatenate Strings("Stop failed with Error Code:0x", w812) -> (w811:string)
                    n579 = One Button Dialog(message=w811) -> ()  [unwired: 2 out]
                  }
                }
              }
            }
          }
        }
      }
      frame "Stiffness calculation" {
        n580 = case shown="\"单线性计算\", 默认" "弯曲计算" {
          tunnel: [w836 w841] -> w834
          tunnel: [w835 w840] -> w833
          tunnel: [w835 w839] -> w832
          tunnel: path "D:/程序文件/弯曲刚度检测数据.txt" ("文件路径输入控件") -> [w837 w838]
          frame "单线性计算", Default {
            n581 = call "弯曲验证.vi"("文件路径输入控件"=w837) -> ("XY图"=w836:cluster{"Y":dbl[], "Y":dbl[]}[], "弯曲刚度值"=w835:dbl)
          }
          frame "弯曲双线性" {
            n582 = call "弯曲双线性曲线图.vi"("文件路径输入控件"=w838) -> ("弯曲刚度值 2"=w839:dbl, "弯曲刚度值1"=w840:dbl, "XY Graph"=w841:cluster{"Y":dbl[], "Y":dbl[]}[])
          }
        }
        "弯曲" <- w834
        "弯曲刚度二" <- w832
        "弯曲刚度一" <- w833
        n583 = call "扭转验证.vi"("文件路径输入控件"=path "D:/程序文件/扭转刚度检测数据.txt") -> ("XY图"=→"扭转":cluster{"Y":dbl[], "Y":dbl[]}[], "扭转刚度值"=→"扭转刚度":dbl)
        n584 = call "拉伸验证.vi"("文件路径输入控件"=path "D:/程序文件/拉伸刚度检测数据.txt") -> ("弯曲刚度值"=→"拉伸刚度":dbl, "XY图"=→"拉伸":cluster{"Y":dbl[], "Y":dbl[]}[])
        n585 = local read "弯曲刚度二"() -> (w823:dbl)
        n586 = local read "扭转刚度"() -> (w821:dbl)
        n587 = local read "拉伸刚度"() -> (w820:dbl)
        n588 = local read "弯曲刚度一"() -> (w822:dbl)
        n589 = Initialize Array(0.0 ("元素"), 2 ("维数大小")) -> (w817:dbl[])
        n590 = Build Array(w823, w822, w821, w820) -> (w815:dbl[])
        n591 = Insert Into Array(array=w817, index=0 ("索引"), new element=w815) -> ()  [unwired: 1 out]
      }
      frame "initialization" {
        w848 = 0.0 ("Position")
        w846 = 0.0 ("Position")
        w847 = 0.0 ("Position")
        n592 = local write "automitic"(FALSE ("automitic")) -> ()
        n593 = call <userlib>:"Acm_GetAvailableDevs.vi"("error in (no error)"=w875) -> ("DeviceList"=w872:T4, "OutEntries"=w871:u32, "error out"=w874:errorcluster)  [unwired: 2 in, 1 out]
        n594 = flat-sequence {
          tunnel: w872 -> [w876]
          tunnel: w871 -> [w877]
          frame #0 {
            n595 = for {
              N: w877 -> [_]
              tunnel: w876 -> [w887] mode=indexing
              tunnel: [w891] -> w879 mode=indexing
              tunnel: [w888] -> w878 mode=indexing
              n596 = Unbundle By Name(w887) -> ("DeviceNum"=w891:u32, "U*8 Array"=w890:T5)  [unwired: 1 out]
              n597 = Cluster To Array(cluster=w890) -> (array=w889:u8[])
              n598 = Byte Array To String(unsigned byte array=w889) -> (string=w888:string)
            }
            "deviceList" <- w879
            n599 = Index Array(array=w879, index="Device Type") -> (element=w882:u32)
            n600 = property on="Device Type" class="Ring (严格)"("Strings []"=w878) -> ()  [unwired: 2 in, 2 out]
            n601 = call <userlib>:"Acm_DevOpen.vi"("DeviceNumber"=w882) -> ("ReturnValue"=w884:u32, "DeviceHandle"=→"DeviceHandle":u32)  [unwired: 1 in, 1 out]
            n602 = Equal?(x=w884, y=u32 0) -> (x = y?=w885:bool)
            "设备打开成功" <- w885
            n603 = Not(x=w885) -> (.not. x?=→"设备关闭成功":bool)
          }
          frame #1 {
            n604 = local read "设备打开成功"() -> (w892:bool)
            n605 = case shown="真" w892 {
              frame False {
              }
              frame True {
                n606 = local read "DeviceHandle"() -> (w895:u32)
                n607 = call <userlib>:"FT_DevAxesCount.vi"("Handle"=w895) -> ("DevAxesCount"=w893:u32)  [unwired: 10 in, 4 out]
                "轴的数量" <- w893
                n608 = for {
                  N: w893 -> [_]
                  tunnel: w895 -> [w899]
                  tunnel: [w898] -> w894 mode=indexing
                  i -> [w900]
                  n609 = call <userlib>:"Acm_AxOpen.vi"("PhyAxis"=w900, "DeviceHandle"=w899) -> ("ReturnValue"=w896:u32, "AxisHandle"=w898:u32)  [unwired: 1 in, 2 out]
                  n610 = Equal To 0?(x=w896) -> (x = 0?=→"轴打开成功":bool)
                }
                "AxisHandle_Array" <- w894
              }
            }
          }
          frame #2 {
            n611 = local read "设备打开成功"() -> (w901:bool)
            n612 = case shown="真" w901 {
              frame False {
              }
              frame True {
                n613 = local read "轴的数量"() -> (w902:u32)
                n614 = for {
                  N: w902 -> [_]
                  i -> [w907]
                  n615 = local read "AxisHandle_Array"() -> (w908:u32[])
                  n616 = Index Array(array=w908, index=w907) -> (element=w906:u32)
                  n617 = call <userlib>:"CFG_AxMaxVel.vi"("CFG_AxMaxVel"=400000.0, "Handle"=w906) -> ("ReturnValue"=w904:u32)  [unwired: 1 in, 2 out]
                  n618 = Equal To 0?(x=w904) -> (x = 0?=→"当前轴达到最大速度":bool)
                }
              }
            }
          }
        }
        n619 = Unbundle By Name(w874) -> ("status"=w873:bool)
        n620 = local write "上行停止状态"(FALSE ("上行停止状态")) -> ()
        n621 = local write "下行状态"(FALSE ("下行状态")) -> ()
        n622 = local write "下行停止状态"(FALSE ("弯曲停止")) -> ()
        n623 = local write "采集卡开关"(FALSE ("采集卡开关")) -> ()
        n624 = local write "上行状态"(FALSE ("上行状态")) -> ()
        n625 = local write "运行状态 2"("initialization" ("运行状态")) -> ()
        n626 = local write "运行状态 3"("initialization" ("运行状态")) -> ()
        n627 = local write "运行状态"("initialization" ("运行状态")) -> ()
        n628 = local write "下行停止状态 2"(FALSE ("下行停止状态")) -> ()
        n629 = local write "下行停止状态 3"(FALSE ("下行停止状态")) -> ()
        n630 = local write "下行状态 2"(FALSE ("下行状态")) -> ()
        n631 = local write "下行状态 3"(FALSE ("下行状态")) -> ()
        n632 = local write "上行停止状态 3"(FALSE ("上行停止状态")) -> ()
        n633 = local write "上行状态 3"(FALSE ("上行状态")) -> ()
        n634 = local write "上行状态 2"(FALSE ("上行状态")) -> ()
        n635 = local write "上行停止状态 2"(FALSE ("上行停止状态")) -> ()
        n636 = local read "AxisHandle_Array"() -> (w857:u32[])
        n637 = local read "AxisHandle_Array"() -> (w854:u32[])
        n638 = local read "AxisHandle_Array"() -> (w853:u32[])
        n639 = Index Array(array=w857, index=4 ("索引")) -> (element=w851:u32)
        n640 = Index Array(array=w854, index=5 ("索引")) -> (element=w850:u32)
        n641 = Index Array(array=w853, index=6 ("索引")) -> (element=w849:u32)
        n642 = call <userlib>:"Acm_AxSetActualPosition.vi"("Position"=w846, "AxisHandle"=w850) -> ()  [unwired: 1 in, 3 out]
        n643 = call <userlib>:"Acm_AxSetActualPosition.vi"("Position"=w847, "AxisHandle"=w851) -> ()  [unwired: 1 in, 3 out]
        n644 = call <userlib>:"Acm_AxSetActualPosition.vi"("Position"=w848, "AxisHandle"=w849) -> ()  [unwired: 1 in, 3 out]
        n645 = local write "拉伸伺服"(w848) -> ()
        n646 = local write "弯曲伺服"(w847) -> ()
        n647 = local write "扭转伺服"(w846) -> ()
      }
      frame "withdraw" {
        n648 = flat-sequence {
          tunnel: [TRUE] -> w909
          frame #0 {
            n649 = local write "采集卡开关"(TRUE ("采集卡开关")) -> ()
            n650 = local write "弯曲控制采集停止状态"(TRUE ("弯曲控制采集")) -> ()
            n651 = local read "AxisHandle_Array"() -> (w926:u32[])
            n652 = Index Array(array=w926, index=6 ("索引")) -> (element=w913:u32)
            n653 = Index Array(array=w926, index=4 ("索引")) -> (element=w919:u32)
            n654 = Index Array(array=w926, index=5 ("索引")) -> (element=w915:u32)
            n655 = call <userlib>:"Acm_AxSetSvOn.vi"("OnOff"=u32 0, "AxisHandle"=w915) -> ()  [unwired: 1 in, 3 out]
            n656 = call <userlib>:"Acm_AxSetSvOn.vi"("OnOff"=u32 0, "AxisHandle"=w913) -> ()  [unwired: 1 in, 3 out]
            n657 = call <userlib>:"Acm_AxSetSvOn.vi"("OnOff"=u32 0, "AxisHandle"=w919) -> ()  [unwired: 1 in, 3 out]
            n658 = call <userlib>:"Acm_AxSetActualPosition.vi"("Position"=0.0, "AxisHandle"=w919) -> ()  [unwired: 1 in, 3 out]
            n659 = call <userlib>:"Acm_AxSetActualPosition.vi"("Position"=0.0, "AxisHandle"=w913) -> ()  [unwired: 1 in, 3 out]
            n660 = call <userlib>:"Acm_AxSetActualPosition.vi"("Position"=0.0, "AxisHandle"=w915) -> ()  [unwired: 1 in, 3 out]
          }
          frame #1 {
            n661 = local read "DeviceHandle"() -> (w935:u32)
            n662 = local write "下行停止状态"(FALSE ("下行停止状态")) -> ()
            n663 = local write "下行状态"(FALSE ("下行状态")) -> ()
            n664 = call <userlib>:"Acm_DevClose.vi"("DeviceHandle"=w935) -> ("ReturnValue"=w927:u32)  [unwired: 1 in, 3 out]
            n665 = local write "上行停止状态"(FALSE ("上行停止状态")) -> ()
            n666 = local write "上行状态"(FALSE ("上行状态")) -> ()
            n667 = Equal To 0?(x=w927) -> (x = 0?=w928:bool)
            n668 = Not(x=w928) -> (.not. x?=w929:bool)
            n669 = case shown="假" w928 {
              tunnel: w927 -> [_ w939]
              frame False {
              }
              frame True {
                n670 = Number To Hexadecimal String(2:w939) -> (0:w937:string)  [unwired: 1 out]
                n671 = Concatenate Strings("Close Board Failed With Error Code:0x", w937) -> (w936:string)
                n672 = One Button Dialog(message=w936) -> ()  [unwired: 2 out]
              }
            }
            n673 = case shown="真" w929 {
              selector: w929 -> [_ w941]
              frame False {
              }
              frame True {
                n674 = local read "轴的数量"() -> (w943:u32)
                n675 = Not(x=w941) -> (.not. x?=w940:bool)
                n676 = local write "轴的数量"(u32 0 ("轴的数量")) -> ()
                n677 = Initialize Array(u32 0 ("元素"), w943) -> (w945:u32[])
                n678 = local write "改变速度成功 2"(w940) -> ()
                n679 = local write "改变速度成功 3"(w940) -> ()
                n680 = local write "急速停止成功 2"(w940) -> ()
                n681 = local write "急速停止成功 3"(w940) -> ()
                n682 = local write "设备打开成功"(w940) -> ()
                n683 = local write "急速停止成功"(w940) -> ()
                n684 = local write "减速停止成功 2"(w940) -> ()
                n685 = local write "减速停止成功 3"(w940) -> ()
                n686 = local write "减速停止成功"(w940) -> ()
                n687 = local write "绝对运动 3"(w940) -> ()
                n688 = local write "绝对运动 2"(w940) -> ()
                n689 = local write "重置计数器成功"(w940) -> ()
                n690 = local write "相对运动 2"(w940) -> ()
                n691 = local write "相对运动 3"(w940) -> ()
                n692 = local write "AxisHandle_Array"(w945) -> ()
                n693 = local write "DeviceHandle"(u32 0 ("DeviceHandle")) -> ()
              }
            }
          }
        }
        n694 = Unbundle By Name(w911) -> ("status"=→"?":bool)
      }
    }
  }
  n695 = while {
    shift-right: [w957] -> _
    shift-left: w15 -> [w960]
    tunnel: w24 -> [w961]
    tunnel: [w954] -> w23
    tunnel: [w953] -> w22
    tunnel: w20 -> [w952]
    tunnel: w17 -> [w951]
    tunnel: w4 -> [w950]
    tunnel: w3 -> [w949]
    tunnel: w6 -> [w948]
    tunnel: w5 -> [w947]
    stop <- w958 stop-if-true
    n696 = register-events(w952, w951, w950, w949, w948, w947) -> (reference out=w955:refnum<event-registration>, error out=w953:errorcluster)  [unwired: 2 in]
    n697 = event shown="[15] \"自动\": 值改变" {
      selector: w955 -> [_ _ _ _ _ _ _ _ _ _ _ _ _ _ _ _ _ _ _ _ _]
      dyn-events: [_ _ _ _ _ _ _ _ _ _ _ _ _ _ _ _ _ _ _ _ _] -> w954
      timeout: _ -> [_ _ _ _ _ _ _ _ _ _ _ _ _ _ _ _ _ _ _ _ _]
      tunnel: w961 -> [w965 w969 w973 w977 w981 w985 w988 w993 w997 w1001 w1005 w1010 w1014 w1018 w1023 w1027 w1031 w1035 w1039 w1044 w1046]
      tunnel: w960 -> [w964 w968 w972 w976 w980 w984 w987 w992 w996 w1000 w1004 w1009 w1013 w1017 w1022 w1026 w1030 w1034 w1038 w1043 w1047]
      tunnel: [w963 w967 w971 w975 w979 w982 w989 w991 w995 w999 w1003 w1008 w1011 w1015 w1021 w1025 w1029 w1033 w1037 w1042 w1047] -> w957
      tunnel: [_ _ _ _ _ _ _ _ _ _ _ _ _ _ _ _ _ _ _ _ "withdraw"] -> w959
      event "弯曲": Value Change {
        n698 = event-data() -> ()  [unwired: 1 in, 1 out]
        n699 = Enqueue Element(queue=w965, element="curve", error in (no error)=w964) -> (error out=w963:errorcluster)  [unwired: 1 in, 2 out]
      }
      event User Event {
        n700 = event-data() -> ()  [unwired: 1 in, 1 out]
        n701 = Enqueue Element(queue=w969, element="Reverse_stop" ("元素"), error in (no error)=w968) -> (error out=w967:errorcluster)  [unwired: 1 in, 2 out]
      }
      event User Event {
        n702 = event-data() -> ()  [unwired: 1 in, 1 out]
        n703 = Enqueue Element(queue=w973, element="reverse_return" ("元素"), error in (no error)=w972) -> (error out=w971:errorcluster)  [unwired: 1 in, 2 out]
      }
      event User Event {
        n704 = event-data() -> ()  [unwired: 1 in, 1 out]
        n705 = Enqueue Element(queue=w977, element="Stretch_stop" ("元素"), error in (no error)=w976) -> (error out=w975:errorcluster)  [unwired: 1 in, 2 out]
      }
      event User Event {
        n706 = event-data() -> ()  [unwired: 1 in, 1 out]
        n707 = Enqueue Element(queue=w981, element="Stretch_return" ("元素"), error in (no error)=w980) -> (error out=w979:errorcluster)  [unwired: 1 in, 2 out]
      }
      event User Event {
        n708 = event-data() -> ()  [unwired: 1 in, 1 out]
        n709 = Enqueue Element(queue=w985, element="Curve_stop" ("元素"), error in (no error)=w984) -> (error out=w982:errorcluster)  [unwired: 1 in, 2 out]
      }
      event User Event {
        n710 = event-data() -> ()  [unwired: 1 in, 1 out]
        n711 = Enqueue Element(queue=w988, element="curve_return" ("元素"), error in (no error)=w987) -> (error out=w989:errorcluster)  [unwired: 1 in, 2 out]
      }
      event "弯曲 2": Value Change {
        n712 = event-data() -> ()  [unwired: 1 in, 1 out]
        n713 = Enqueue Element(queue=w993, element="curve2" ("元素"), error in (no error)=w992) -> (error out=w991:errorcluster)  [unwired: 1 in, 2 out]
      }
      event "刚度计算": Value Change {
        n714 = event-data() -> ()  [unwired: 1 in, 1 out]
        n715 = Enqueue Element(queue=w997, element="Stiffness calculation" ("元素"), error in (no error)=w996) -> (error out=w995:errorcluster)  [unwired: 1 in, 2 out]
      }
      event "扭转": Value Change {
        n716 = event-data() -> ()  [unwired: 1 in, 1 out]
        n717 = Enqueue Element(queue=w1001, element="Reverse" ("元素"), error in (no error)=w1000) -> (error out=w999:errorcluster)  [unwired: 1 in, 2 out]
      }
      event "复位2": Value Change {
        n718 = event-data() -> ()  [unwired: 1 in, 1 out]
        n719 = Enqueue Element(queue=w1005, element="reset2" ("元素"), error in (no error)=w1004) -> (error out=w1003:errorcluster)  [unwired: 1 in, 2 out]
      }
      event "停止2": Value Change {
        n720 = event-data() -> ()  [unwired: 1 in, 1 out]
        n721 = Enqueue Element(queue=w1010, element="stop2" ("元素"), error in (no error)=w1009) -> (error out=w1008:errorcluster)  [unwired: 1 in, 2 out]
        "扭转停止" <- TRUE ("扭转停止")
      }
      event "拉伸": Value Change {
        n722 = event-data() -> ()  [unwired: 1 in, 1 out]
        n723 = Enqueue Element(queue=w1014, element="Stretch" ("元素"), error in (no error)=w1013) -> (error out=w1011:errorcluster)  [unwired: 1 in, 2 out]
      }
      event "复位3": Value Change {
        n724 = event-data() -> ()  [unwired: 1 in, 1 out]
        n725 = Enqueue Element(queue=w1018, element="reset3" ("元素"), error in (no error)=w1017) -> (error out=w1015:errorcluster)  [unwired: 1 in, 2 out]
      }
      event "停止3": Value Change {
        n726 = event-data() -> ()  [unwired: 1 in, 1 out]
        n727 = Enqueue Element(queue=w1023, element="stop3" ("元素"), error in (no error)=w1022) -> (error out=w1021:errorcluster)  [unwired: 1 in, 2 out]
        "拉伸停止" <- TRUE ("拉伸停止")
      }
      event "自动": Value Change {
        n728 = event-data() -> ()  [unwired: 1 in, 1 out]
        n729 = Enqueue Element(queue=w1027, element="automatic" ("元素"), error in (no error)=w1026) -> (error out=w1025:errorcluster)  [unwired: 1 in, 2 out]
      }
      event "手动": Mouse Down {
        n730 = event-data() -> ()  [unwired: 1 in, 1 out]
        n731 = Enqueue Element(queue=w1031, element="manual control" ("元素"), error in (no error)=w1030) -> (error out=w1029:errorcluster)  [unwired: 1 in, 2 out]
      }
      event "手动": Mouse Leave {
        n732 = event-data() -> ()  [unwired: 1 in, 1 out]
        n733 = Enqueue Element(queue=w1035, element="stop3_leave" ("元素"), error in (no error)=w1034) -> (error out=w1033:errorcluster)  [unwired: 1 in, 2 out]
      }
      event "复位1": Value Change {
        n734 = event-data() -> ()  [unwired: 1 in, 1 out]
        n735 = Enqueue Element(queue=w1039, element="reset1" ("元素"), error in (no error)=w1038) -> (error out=w1037:errorcluster)  [unwired: 1 in, 2 out]
      }
      event "停止1": Value Change {
        n736 = event-data() -> ()  [unwired: 1 in, 1 out]
        n737 = Enqueue Element(queue=w1044, element="stop1" ("元素"), error in (no error)=w1043) -> (error out=w1042:errorcluster)  [unwired: 1 in, 2 out]
        "弯曲停止" <- TRUE ("弯曲停止")
      }
      event "withdraw": Value Change {
        n738 = event-data() -> ()  [unwired: 1 in, 1 out]
        n739 = Enqueue Element(queue=w1046, element="withdraw" ("元素")) -> ()  [unwired: 2 in, 3 out]
      }
    }
    n740 = Unbundle By Name(w957) -> ("status"=w956:bool)
    n741 = Or(x=w956, y=w959) -> (x .or. y?=w958:bool)
  }
  n742 = Unregister For Events(event registration refnum=w23, error in=w22) -> (error out=w1:errorcluster)
  n743 = Release Queue(queue=w24, error in (no error)=w1) -> (error out=w2:errorcluster)  [unwired: 1 in, 2 out]
  n744 = Destroy User Event(user event=w20, error in=w2) -> (error out=w18:errorcluster)
  n745 = Destroy User Event(user event=w17, error in=w18) -> (error out=w9:errorcluster)
  n746 = Destroy User Event(user event=w4, error in=w9) -> (error out=w10:errorcluster)
  n747 = Destroy User Event(user event=w3, error in=w10) -> (error out=w8:errorcluster)
  n748 = Destroy User Event(user event=w6, error in=w8) -> (error out=w7:errorcluster)
  n749 = Destroy User Event(user event=w5, error in=w7) -> ()  [unwired: 1 out]
  "弯曲控制采集停止状态" <- FALSE ("弯曲控制采集")
